vi "Main.vi"() -> ()   [LabVIEW 2013]
uses:
  <vilib>/Utility/error.llb/DialogType.ctl
  <vilib>/Utility/miscctls.llb/LVFontTypeDef.ctl
panel:
  in  "List of channels":i32(listbox)
  in  "ReadFromFile":bool
  in  "WriteToFile":bool
  out "Дата":string
  out "Время":string
  in  "Comm. current inc":dbl=0.5 caption="А" min=0.0 max=72.0 step=0.25
  in  "Common curr. dec":bool
  in  "Common curr. inc":bool
  in  "ConnectAll":bool
  in  "DisconnectAll":bool
  in  "Set Output ON All":bool caption="ВЫХОДЫ ИСТОЧНИКОВ"
  out "текущий ист.":u8
  in  "SetCurrent":dbl min=0.0 max=72.0 step=0.1 format="%#.1g"
  in  "SetVoltage":dbl min=0.0 max=30.0 step=0.1 format="%#.1g"
  in  "SetCurrentB":bool
  in  "SetVoltageB":bool
  in  "SetOutputOffB":bool
  in  "SetOutputOnB":bool
  in  "ConnectChannel":bool
  in  "DisconnectChannel":bool
  in  "stop":bool
  out "Buv con ID":refnum<k5>
  out "LoadPhase":bool
  in  "SetCurrentAll":bool
  in  "SetVoltageAll":bool
  in  "Comm. voltage %":dbl caption="%" min=0.0 max=100.0 step=0.5
  in  "Common volt. dec":bool
  in  "Common volt. inc":bool
  in  "DeleteChannel":bool
  in  "AddChannel":bool
  out "CURRENTSET":dbl[](array[numeric])
  out "NAME":string[](array[string])
  out "ADRESS":string[](array[string])
  out "Measure_VI":refnum<vi>[](array[refnum])
  # "ЛИНЗЫ ЖЕСТКОЙ ФОКУСИРОВКИ ПОСТОЯННОГО ТОКА"
  # "ВСЕ ИСТОЧНИКИ"
  # "ИСТОЧНИК №_"
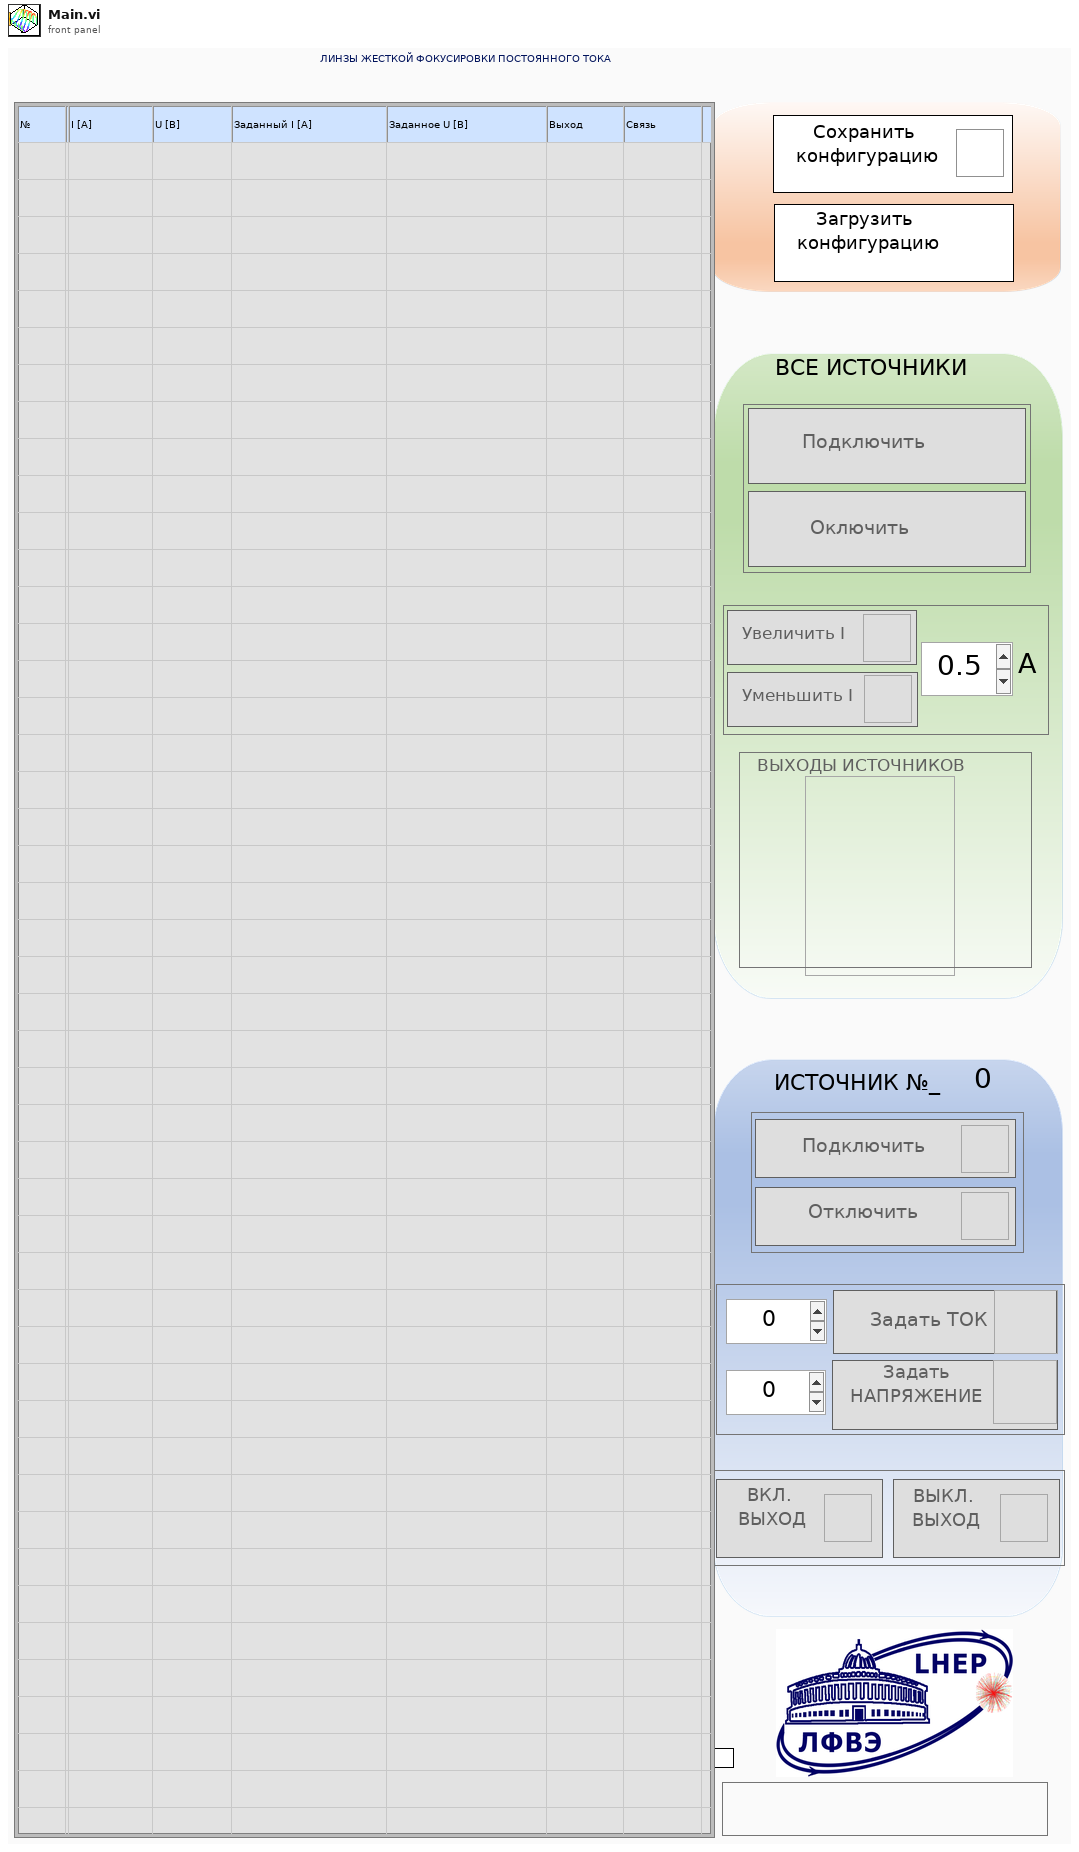
[diagram p1: front panel]
types:
  T1 = enum8{"Enabled", "Disabled", "Disabled and Grayed Out"}
  T2 = enum16{"open", "replace", "create", "open or create", "replace or create", "replace or create with confirmation"}
  T3 = typedef "DialogType.ctl" = u16
  T4 = typedef "LVFontTypeDef.ctl" = cluster{"Font Name":string, "Size":u16, "Bold":bool, "Italic":bool, "Underline":bool, "Strikeout":bool, "Color":u32}
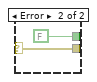
[diagram p7: hidden frame]
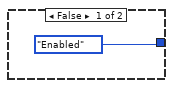
[diagram p9: hidden frame]
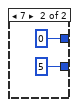
[diagram p11: hidden frame]
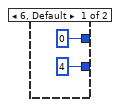
[diagram p12: hidden frame]
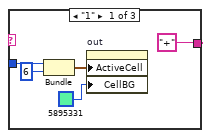
[diagram p13: hidden frame]
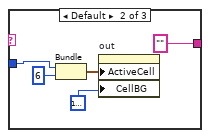
[diagram p14: hidden frame]
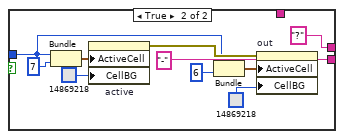
[diagram p15: hidden frame]
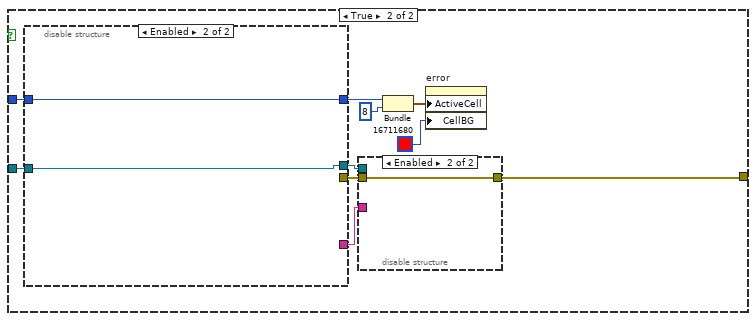
[diagram p16: hidden frame]
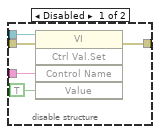
[diagram p17: hidden frame]
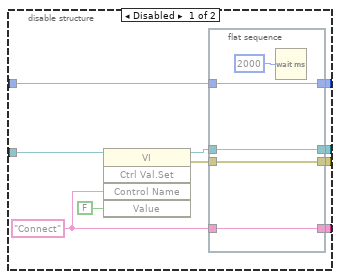
[diagram p18: hidden frame]
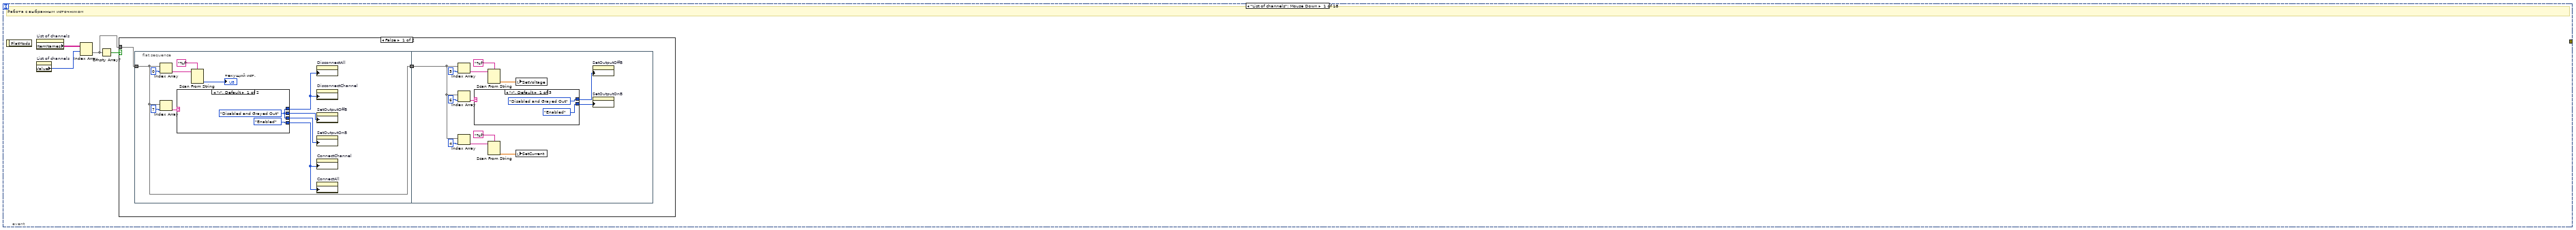
[diagram p19: hidden frame]
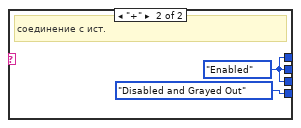
[diagram p20: hidden frame]
diagram:
  w1 = string[] [] ("GlobalInAdress")
  (unwired) T1."Enabled" ("Disabled")
  w17 = u8 0 ("Disabled")
  w4 = FALSE ("SetOutputOnB")
  n1 = while {
    stop <- FALSE stop-if-true
    n2 = property on="List of channels" class="MCListbox (strict)"() -> ("ItemNames"=w29:string[][])  [unwired: 2 in, 2 out]
    n3 = Get Date/Time String(want seconds? (F)=TRUE) -> (date string=→"Дата":string, time string=→"Время":string)  [unwired: 2 in]
    n4 = Wait Until Next ms Multiple(millisecond multiple=u16 1000) -> ()  [unwired: 1 out]
    n5 = Empty Array?(array=w29) -> (empty?=w28:bool)
    n6 = case shown="True" w28 {
      tunnel: [T1."Enabled" ("Disabled") T1."Disabled and Grayed Out" ("Disabled")] -> w23
      frame False {
      }
      frame True {
      }
    }
    n7 = property on="Common curr. inc" class="Bool (strict)"("DisabledEnum"=w23) -> ()  [unwired: 2 in, 2 out]
    n8 = property on="Common curr. dec" class="Bool (strict)"("DisabledEnum"=w23) -> ()  [unwired: 2 in, 2 out]
    n9 = property on="Set Output ON All" class="Bool (strict)"("DisabledEnum"=w23) -> ()  [unwired: 2 in, 2 out]
    n10 = property on="Common volt. inc" class="Bool (strict)"("DisabledEnum"=w23) -> ()  [unwired: 2 in, 2 out]
    n11 = property on="DisconnectAll" class="Bool (strict)"("DisabledEnum"=w23) -> ()  [unwired: 2 in, 2 out]
    n12 = property on="SetVoltageB" class="Bool (strict)"("DisabledEnum"=w23) -> ()  [unwired: 2 in, 2 out]
    n13 = property on="ConnectChannel" class="Bool (strict)"("DisabledEnum"=w23) -> ()  [unwired: 2 in, 2 out]
    n14 = property on="SetOutputOnB" class="Bool (strict)"("DisabledEnum"=w23) -> ()  [unwired: 2 in, 2 out]
    n15 = property on="DisconnectChannel" class="Bool (strict)"("DisabledEnum"=w23) -> ()  [unwired: 2 in, 2 out]
    n16 = property on="SetOutputOffB" class="Bool (strict)"("DisabledEnum"=w23) -> ()  [unwired: 2 in, 2 out]
    n17 = property on="ConnectAll" class="Bool (strict)"("DisabledEnum"=w23) -> ()  [unwired: 2 in, 2 out]
    n18 = property on="SetCurrentB" class="Bool (strict)"("DisabledEnum"=w23) -> ()  [unwired: 2 in, 2 out]
  }
  n19 = while {
    stop <- FALSE stop-if-true
    n20 = property on="AddChannel" class="Bool (strict)"() -> ("Disabled"=w37:u8)  [unwired: 2 in, 2 out]
    n21 = Wait Until Next ms Multiple(millisecond multiple=u32 10) -> ()  [unwired: 1 out]
    n22 = Equal?(x=w37, y=u8 0) -> (x = y?=w33:bool)
    n23 = case shown="True" w33 {
      frame False {
      }
      frame True {
        w43 = string[] [] ("GlobalInAdress")
        n24 = local read "Measure_VI"() -> (w50:refnum<vi>[])
        n25 = Array Size(array=w50) -> (size(s)=w42:i32)
        n26 = for {
          N: w42 -> [_]
          tunnel: w50 -> [w113]
          shift-right: [w55] -> w41
          shift-left: w43 -> [w52]
          shift-right: [w54] -> w40
          shift-left: w43 -> [w53]
          shift-right: [w104] -> w38
          shift-left: w43 -> [w105]
          shift-right: [w95] -> w39
          shift-left: w43 -> [w100]
          shift-right: [w98] -> w46
          shift-left: w43 -> [w80]
          shift-right: [w93] -> w45
          shift-left: w43 -> [w94]
          i -> [w76]
          w92 = "" ("Control Name")
          n27 = Index Array(array=w113, index=w76) -> (element=w79:refnum<vi>)
          n28 = invoke on="Invoke Node" class="VI" method="Ctrl Val.Get"(reference=w79, "Control Name"="SetVoltageStr") -> (error out=w87:errorcluster, "Get Control Value Variant"=w103:variant)  [unwired: 2 in, 2 out]
          n29 = invoke class="VI" method="Ctrl Val.Get"(reference=w79, "Control Name"="SetCurrentStr") -> (error out=w86:errorcluster, "Get Control Value Variant"=w102:variant)  [unwired: 2 in, 2 out]
          n30 = invoke class="VI" method="Ctrl Val.Get"(reference=w79, "Control Name"="Error") -> (error out=w75:errorcluster, "Get Control Value Variant"=w81:variant)  [unwired: 2 in, 2 out]
          n31 = invoke class="VI" method="Ctrl Val.Get"(reference=w79, "Control Name"="GetCurrent") -> (error out=w89:errorcluster, "Get Control Value Variant"=w110:variant)  [unwired: 2 in, 2 out]
          n32 = invoke class="VI" method="Ctrl Val.Get"(reference=w79, "Control Name"="GetVoltage") -> (error out=w88:errorcluster, "Get Control Value Variant"=w111:variant)  [unwired: 2 in, 2 out]
          n33 = invoke class="VI" method="Ctrl Val.Get"(reference=w79, "Control Name"="Output") -> (error out=w85:errorcluster, "Get Control Value Variant"=w96:variant)  [unwired: 2 in, 2 out]
          n34 = Variant To Data(type=w92, Variant=w103) -> (data=w57:string)  [unwired: 1 in, 1 out]
          n35 = Variant To Data(type=w92, Variant=w102) -> (data=w62:string)  [unwired: 1 in, 1 out]
          n36 = Merge Errors(w75, w89, w88, w87) -> (w84:errorcluster)
          n37 = Variant To Data(type=w92, Variant=w110) -> (data=w107:string)  [unwired: 1 in, 1 out]
          n38 = Variant To Data(type=w92, Variant=w111) -> (data=w108:string)  [unwired: 1 in, 1 out]
          n39 = Variant To Data "Out"(type=w92, Variant=w96) -> (data=w82:string)  [unwired: 1 in, 1 out]
          n40 = Merge Errors(w86, w85) -> (w83:errorcluster)
          n41 = String Length(string=w57) -> (length=w58:i32)
          n42 = String Length(string=w62) -> (length=w65:i32)
          n43 = Variant To Data(type=FALSE, Variant=w81) -> (data=w51:bool)  [unwired: 1 in, 1 out]
          n44 = case shown="False" w51 {
            tunnel: w79 -> [_ w167]
            tunnel: w76 -> [w154 w160]
            tunnel: [w153 w158] -> w72
            frame False {
              n45 = Bundle(w154, "milliseconds to wait"=8) -> (w155:cluster{i32, "milliseconds to wait":i32})  [unwired: 1 in]
              n46 = property on="error" class="MCListbox (strict)"("ActiveCell"=w155, "CellBG"=u32 16777225) -> (error out=w153:errorcluster)  [unwired: 2 in, 1 out]
            }
            frame True {
              n47 = disable-structure shown="Enabled" {
                disable-tunnel: w167 -> [w183 w189]
                disable-tunnel: [w180 _] -> w163
                disable-tunnel: [w178 w189] -> w162
                disable-tunnel: [w176 _] -> w161
                disable-tunnel: w160 -> [w175 w190]
                disable-tunnel: [w174 w190] -> w159
                frame Disabled {
                  w177 = "Connect" ("Control Name")
                  n48 = invoke class="VI" method="Ctrl Val.Set"(reference=w183, "Control Name"=w177, "Value"=FALSE ("OK Button")) -> (reference out=w179:refnum<vi>, error out=w181:errorcluster)  [unwired: 2 in, 3 out]
                  n49 = flat-sequence {
                    tunnel: w181 -> [w188]
                    tunnel: [w188] -> w180
                    tunnel: w179 -> [w186]
                    tunnel: [w186] -> w178
                    tunnel: w177 -> [w185]
                    tunnel: [w185] -> w176
                    tunnel: w175 -> [w184]
                    tunnel: [w184] -> w174
                    frame #0 {
                      n50 = Wait (ms)(milliseconds to wait=u32 2000) -> ()  [unwired: 1 out]
                    }
                  }
                }
                frame Enabled {
                }
              }
              n51 = disable-structure shown="Enabled" {
                disable-tunnel: w163 -> [w171 w173]
                disable-tunnel: w162 -> [w170 _]
                disable-tunnel: w161 -> [w169 _]
                disable-tunnel: [w168 w173] -> w158
                frame Disabled {
                  n52 = invoke class="VI" method="Ctrl Val.Set"(reference=w170, error in=w171, "Control Name"=w169, "Value"=TRUE ("OK Button")) -> (error out=w168:errorcluster)  [unwired: 1 in, 4 out]
                }
                frame Enabled {
                }
              }
              n53 = Bundle(w159, "milliseconds to wait"=8) -> (w164:cluster{i32, "milliseconds to wait":i32})  [unwired: 1 in]
              n54 = property on="error" class="MCListbox (strict)"("ActiveCell"=w164, "CellBG"=u32 16711680) -> ()  [unwired: 2 in, 2 out]
            }
          }
          n55 = case shown="6, Default" w58 {
            tunnel: [4 ("milliseconds to wait") 5 ("milliseconds to wait")] -> w59
            tunnel: [0 ("milliseconds to wait") 0 ("milliseconds to wait")] -> w60
            frame 6, Default {
            }
            frame 7 {
            }
          }
          n56 = case shown="7" w65 {
            tunnel: [4 ("milliseconds to wait") 5 ("milliseconds to wait")] -> w64
            tunnel: [0 ("milliseconds to wait") 0 ("milliseconds to wait")] -> w63
            frame 6, Default {
            }
            frame 7 {
            }
          }
          n57 = Build Array (concatenate)(w52, w107) -> (w55:string[])
          n58 = Build Array (concatenate)(w53, w108) -> (w54:string[])
          n59 = Merge Errors(w84, w83, w72) -> (w78:errorcluster)
          n60 = call <vilib>:"General Error Handler.vi"("type of dialog (OK msg:1)"=u32 0 ("milliseconds to wait"), "error in (no error)"=w78) -> ()  [unwired: 9 in, 5 out]
          n61 = case shown="\"0\"" w82 {
            tunnel: ["+" ("Control Name") "" ("Control Name") "-" ("Control Name")] -> w74
            tunnel: w76 -> [w122 w127 w132]
            frame "1" {
              n62 = Bundle(w122, "milliseconds to wait"=6) -> (w124:cluster{i32, "milliseconds to wait":i32})  [unwired: 1 in]
              n63 = property on="out" class="MCListbox (strict)"("ActiveCell"=w124, "CellBG"=u32 5895331) -> ()  [unwired: 2 in, 2 out]
            }
            frame Default {
              n64 = Bundle(w127, "milliseconds to wait"=6) -> (w129:cluster{i32, "milliseconds to wait":i32})  [unwired: 1 in]
              n65 = property on="out" class="MCListbox (strict)"("ActiveCell"=w129, "CellBG"=u32 16777225) -> ()  [unwired: 2 in, 2 out]
            }
            frame "0" {
              n66 = Bundle(w132, "milliseconds to wait"=6) -> (w134:cluster{i32, "milliseconds to wait":i32})  [unwired: 1 in]
              n67 = property on="out" class="MCListbox (strict)"("ActiveCell"=w134, "CellBG"=u32 13816530) -> ()  [unwired: 2 in, 2 out]
            }
          }
          n68 = String Subset(string=w57, offset (0)=w60, length (rest)=w59) -> (substring=w56:string)
          n69 = String Subset(string=w62, offset (0)=w63, length (rest)=w64) -> (substring=w61:string)
          n70 = case shown="False" w51 {
            tunnel: ["+" ("Control Name") "-" ("Control Name")] -> w99
            tunnel: w76 -> [w138 w145]
            tunnel: w74 -> [w137 _]
            tunnel: [w137 "?" ("Control Name")] -> w73
            frame False {
              n71 = Bundle(w138, "milliseconds to wait"=7) -> (w140:cluster{i32, "milliseconds to wait":i32})  [unwired: 1 in]
              n72 = property on="active" class="MCListbox (strict)"("ActiveCell"=w140, "CellBG"=u32 5895331) -> ()  [unwired: 2 in, 2 out]
            }
            frame True {
              n73 = Bundle(w145, "milliseconds to wait"=7) -> (w151:cluster{i32, "milliseconds to wait":i32})  [unwired: 1 in]
              n74 = property on="active" class="MCListbox (strict)"("ActiveCell"=w151, "CellBG"=u32 14869218) -> (error out=w146:errorcluster)  [unwired: 2 in, 1 out]
              n75 = Bundle(w145, "milliseconds to wait"=6) -> (w144:cluster{i32, "milliseconds to wait":i32})  [unwired: 1 in]
              n76 = property on="out" class="MCListbox (strict)"(error in=w146, "ActiveCell"=w144, "CellBG"=u32 14869218) -> ()  [unwired: 1 in, 2 out]
            }
          }
          n77 = Search and Replace String(input string=w56, search string=",", replace string="." ("replace string (\"\")")) -> (result string=w69:string)  [unwired: 5 in, 3 out]
          n78 = Search and Replace String(input string=w61, search string=",", replace string="." ("replace string (\"\")")) -> (result string=w67:string)  [unwired: 5 in, 3 out]
          n79 = Build Array (concatenate)(w100, w67) -> (w95:string[])
          n80 = Build Array (concatenate)(w105, w69) -> (w104:string[])
          n81 = Build Array (concatenate)(w94, w73) -> (w93:string[])
          n82 = Build Array (concatenate)(w80, w99) -> (w98:string[])
        }
        n83 = local read "ADRESS"() -> (w48:string[])
        n84 = local read "NAME"() -> (w47:string[])
        n85 = Build Array(w47, w48, w41, w40, w39, w38, w45, w46) -> (w49:string[][])
        n86 = Transpose 2D Array(2D array=w49) -> (transposed array=w44:string[][])
        n87 = property on="List of channels" class="MCListbox (strict)"("ItemNames"=w44) -> ()  [unwired: 2 in, 2 out]
      }
    }
  }
  n88 = while {
    stop <- FALSE stop-if-true
    n89 = event shown="[11] \"SetOutputOnB\": Value Change" {
      selector: _ -> [_ _ _ _ _ _ _ _ _ _ _ _ _ _ _ _ _ _]
      dyn-events: _ -> [_ _ _ _ _ _ _ _ _ _ _ _ _ _ _ _ _ _]
      timeout: _ -> [_ _ _ _ _ _ _ _ _ _ _ _ _ _ _ _ _ _]
      tunnel: [_ _ w261 w277 w293 w334 w375 w390 w421 w437 w453 w470 w491 w514 w532 w583 w661 w684] -> w192
      event "List of channels": Mouse Down {
        # "Работа с выбранным источником"
        n90 = event-data() -> ()  [unwired: 2 out]
        n91 = property on="List of channels" class="MCListbox (strict)"() -> ("ItemNames"=w198:string[][])  [unwired: 2 in, 2 out]
        n92 = property on="List of channels" class="MCListbox (strict)"() -> ("Value"=w197:i32)  [unwired: 2 in, 2 out]
        n93 = Index Array(array=w198, index (row)=w197) -> (element=w196:string[])  [unwired: 1 in]
        n94 = Empty Array?(array=w196) -> (empty?=w195:bool)
        n95 = case shown="False" w195 {
          tunnel: w196 -> [w199 _]
          frame False {
            n96 = flat-sequence {
              tunnel: w199 -> [w205]
              tunnel: [w205] -> w200
              tunnel: w200 -> [w218]
              frame #0 {
                n97 = Index Array(array=w205, index=0) -> (element=w208:string)
                n98 = Index Array(array=w205, index=7) -> (element=w206:string)
                n99 = case shown="\"-\", Default" w206 {
                  tunnel: [T1."Enabled" ("Disabled") T1."Disabled and Grayed Out" ("Disabled")] -> w201
                  tunnel: [w212 w214] -> w202
                  tunnel: [w212 w214] -> w204
                  tunnel: [w212 w214] -> w203
                  frame "-", Default {
                    w212 = T1."Disabled and Grayed Out" ("Disabled")
                  }
                  frame "+" {
                    w214 = T1."Enabled" ("Disabled")
                    # "соединение с ист."
                  }
                }
                n100 = Scan From String(format string="%f", input string=w208) -> (output 1=→"текущий ист.":u8)  [unwired: 3 in, 3 out]
                n101 = property on="DisconnectAll" class="Bool (strict)"("DisabledEnum"=w202) -> ()  [unwired: 2 in, 2 out]
                n102 = property on="DisconnectChannel" class="Bool (strict)"("DisabledEnum"=w202) -> ()  [unwired: 2 in, 2 out]
                n103 = property on="SetOutputOffB" class="Bool (strict)"("DisabledEnum"=w204) -> ()  [unwired: 2 in, 2 out]
                n104 = property on="SetOutputOnB" class="Bool (strict)"("DisabledEnum"=w203) -> ()  [unwired: 2 in, 2 out]
                n105 = property on="ConnectChannel" class="Bool (strict)"("DisabledEnum"=w201) -> ()  [unwired: 2 in, 2 out]
                n106 = property on="ConnectAll" class="Bool (strict)"("DisabledEnum"=w201) -> ()  [unwired: 2 in, 2 out]
              }
              frame #1 {
                n107 = Index Array(array=w218, index=5) -> (element=w223:string)
                n108 = Index Array(array=w218, index=6) -> (element=w226:string)
                n109 = Index Array(array=w218, index=4) -> (element=w220:string)
                n110 = case shown="\"-\", Default" w226 {
                  tunnel: [T1."Enabled" ("Disabled") T1."Disabled and Grayed Out" ("Disabled") w233] -> w227
                  tunnel: [T1."Disabled and Grayed Out" ("Disabled") T1."Enabled" ("Disabled") w233] -> w228
                  frame "-", Default {
                  }
                  frame "+" {
                  }
                  frame "?" {
                    w233 = T1."Disabled and Grayed Out" ("Disabled")
                  }
                }
                n111 = Scan From String(format string="%f", input string=w223) -> (output 1=w216:dbl)  [unwired: 3 in, 3 out]
                n112 = Scan From String(format string="%f", input string=w220) -> (output 1=w217:dbl)  [unwired: 3 in, 3 out]
                n113 = local write "SetVoltage"(w216) -> ()
                n114 = local write "SetCurrent"(w217) -> ()
                n115 = property on="SetOutputOffB" class="Bool (strict)"("DisabledEnum"=w228) -> ()  [unwired: 2 in, 2 out]
                n116 = property on="SetOutputOnB" class="Bool (strict)"("DisabledEnum"=w227) -> ()  [unwired: 2 in, 2 out]
              }
            }
          }
          frame True {
          }
        }
      }
      event Panel Close? {
        n117 = event-data() -> ()  [unwired: 5 out]
        n118 = Two Button Dialog(message="Вы уверены, что хотите закрыть программу?", 1:"Нет" ("F button name (\"Cancel\")"), 2:"Да" ("T button name (\"OK\")")) -> (T button?=w237:bool)
        n119 = case shown="True" w237 {
          frame False {
          }
          frame True {
            n120 = disable-structure shown="Disabled" {
              frame Disabled {
                n121 = local read item#-1() -> (w247)
                n122 = TCP Close Connection(connection ID=w247) -> ()  [unwired: 2 in, 2 out]
              }
              frame Enabled {
              }
            }
            n123 = local read "Measure_VI"() -> (w239:refnum<vi>[])
            n124 = Array Size(array=w239) -> (size(s)=w238:i32)
            n125 = for {
              N: w238 -> [_]
              tunnel: w239 -> [w257]
              tunnel: [w255] -> w246 mode=indexing
              i -> [w258]
              n126 = Index Array(array=w257, index=w258) -> (element=w256:refnum<vi>)
              n127 = invoke class="VI" method="Ctrl Val.Set"(reference=w256, "Control Name"="Connect", "Value"=FALSE) -> (error out=w255:errorcluster)  [unwired: 2 in, 4 out]
            }
            n128 = flat-sequence {
              tunnel: [w249] -> w245
              tunnel: w246 -> [w249]
              frame #0 {
                n129 = Wait (ms)(milliseconds to wait=u32 1000) -> ()  [unwired: 1 out]
              }
            }
            n130 = local read "Measure_VI"() -> (w240:refnum<vi>[])
            n131 = Array Size(array=w240) -> (size(s)=w241:i32)
            n132 = for {
              N: w241 -> [_]
              tunnel: w240 -> [w253]
              tunnel: [w251] -> w242 mode=indexing
              tunnel: w245 -> [w250] mode=indexing
              i -> [w254]
              n133 = Index Array(array=w253, index=w254) -> (element=w252:refnum<vi>)
              n134 = invoke class="VI" method="Abort VI"(reference=w252, error in=w250) -> (error out=w251:errorcluster)  [unwired: 1 in, 2 out]
            }
            n135 = Merge Errors(w242) -> (w243:errorcluster)
            n136 = call <vilib>:"General Error Handler.vi"("type of dialog (OK msg:1)"=u32 0 ("milliseconds to wait"), "error in (no error)"=w243) -> ()  [unwired: 9 in, 5 out]
          }
        }
        n137 = event-data() -> ()  [unwired: 2 in, 1 out]
      }
      event "SetVoltageAll": Value Change {
        n138 = event-data() -> ()  [unwired: 7 out]
        n139 = flat-sequence {
          tunnel: [w265] -> w263
          tunnel: [w274] -> w262
          tunnel: w263 -> [w274]
          frame #0 {
            w264 = u8 2 ("Disabled")
            n140 = property on="AddChannel" class="Bool (strict)"("Disabled"=w264) -> ()  [unwired: 2 in, 2 out]
            n141 = property on="DisconnectChannel" class="Bool (strict)"("Disabled"=w264) -> ()  [unwired: 2 in, 2 out]
            n142 = property on="ConnectAll" class="Bool (strict)"("Disabled"=w264) -> ()  [unwired: 2 in, 2 out]
            n143 = property on="ReadFromFile" class="Bool (strict)"("Disabled"=w264) -> ()  [unwired: 2 in, 2 out]
            n144 = property on="ConnectChannel" class="Bool (strict)"("Disabled"=w264) -> ()  [unwired: 2 in, 2 out]
            n145 = property on="DeleteChannel" class="Bool (strict)"("Disabled"=w264) -> ()  [unwired: 2 in, 2 out]
            n146 = property on="SetVoltageB" class="Bool (strict)"("Disabled"=w264) -> ()  [unwired: 2 in, 2 out]
            n147 = property on="Set Output ON All" class="Bool (strict)"("Disabled"=w264) -> ()  [unwired: 2 in, 2 out]
            n148 = property on="SetOutputOffB" class="Bool (strict)"("Disabled"=w264) -> ()  [unwired: 2 in, 2 out]
            n149 = property on="SetVoltageAll" class="Bool (strict)"("Disabled"=w264) -> ()  [unwired: 2 in, 2 out]
            n150 = property on="SetCurrentAll" class="Bool (strict)"("Disabled"=w264) -> ()  [unwired: 2 in, 2 out]
            n151 = property on="DisconnectAll" class="Bool (strict)"("Disabled"=w264) -> ()  [unwired: 2 in, 2 out]
            n152 = property on="WriteToFile" class="Bool (strict)"("Disabled"=w264) -> ()  [unwired: 2 in, 2 out]
            n153 = property on="SetCurrentB" class="Bool (strict)"("Disabled"=w264) -> ()  [unwired: 2 in, 2 out]
            n154 = property on="SetOutputOnB" class="Bool (strict)"("Disabled"=w264) -> ()  [unwired: 2 in, 2 out]
          }
          frame #1 {
            n155 = local read "Measure_VI"() -> (w267:refnum<vi>[])
            n156 = Array Size(array=w267) -> (size(s)=w266:i32)
            n157 = for {
              N: w266 -> [_]
              tunnel: [w268] -> w265 mode=indexing
              i -> [w270]
              n158 = local read "Measure_VI"() -> (w273:refnum<vi>[])
              n159 = Index Array(array=w273, index=w270) -> (element=w269:refnum<vi>)
              n160 = invoke class="VI" method="Ctrl Val.Set"(reference=w269, "Control Name"="NeedToSetVoltage", "Value"=TRUE ("ConnectChannel")) -> (error out=w268:errorcluster)  [unwired: 2 in, 4 out]
            }
          }
          frame #2 {
            w275 = u8 0 ("Disabled")
            n161 = local write "SetVoltageAll"(FALSE ("SetVoltageAll")) -> ()
            n162 = property on="AddChannel" class="Bool (strict)"("Disabled"=w275) -> ()  [unwired: 2 in, 2 out]
            n163 = property on="DisconnectChannel" class="Bool (strict)"("Disabled"=w275) -> ()  [unwired: 2 in, 2 out]
            n164 = property on="ReadFromFile" class="Bool (strict)"("Disabled"=w275) -> ()  [unwired: 2 in, 2 out]
            n165 = property on="ConnectChannel" class="Bool (strict)"("Disabled"=w275) -> ()  [unwired: 2 in, 2 out]
            n166 = property on="DeleteChannel" class="Bool (strict)"("Disabled"=w275) -> ()  [unwired: 2 in, 2 out]
            n167 = property on="WriteToFile" class="Bool (strict)"("Disabled"=w275) -> ()  [unwired: 2 in, 2 out]
            n168 = property on="Set Output ON All" class="Bool (strict)"("Disabled"=w275) -> ()  [unwired: 2 in, 2 out]
            n169 = property on="SetCurrentB" class="Bool (strict)"("Disabled"=w275) -> ()  [unwired: 2 in, 2 out]
            n170 = property on="ConnectAll" class="Bool (strict)"("Disabled"=w275) -> ()  [unwired: 2 in, 2 out]
            n171 = property on="SetOutputOnB" class="Bool (strict)"("Disabled"=w275) -> ()  [unwired: 2 in, 2 out]
            n172 = property on="SetVoltageB" class="Bool (strict)"("Disabled"=w275) -> ()  [unwired: 2 in, 2 out]
            n173 = property on="SetOutputOffB" class="Bool (strict)"("Disabled"=w275) -> ()  [unwired: 2 in, 2 out]
            n174 = property on="SetVoltageAll" class="Bool (strict)"("Disabled"=w275) -> ()  [unwired: 2 in, 2 out]
            n175 = property on="SetCurrentAll" class="Bool (strict)"("Disabled"=w275) -> ()  [unwired: 2 in, 2 out]
            n176 = property on="DisconnectAll" class="Bool (strict)"("Disabled"=w275) -> ()  [unwired: 2 in, 2 out]
          }
        }
        n177 = Merge Errors(w262) -> (w261:errorcluster)
      }
      event "SetCurrentAll": Value Change {
        n178 = event-data() -> ()  [unwired: 7 out]
        n179 = flat-sequence {
          tunnel: [w281] -> w279
          tunnel: [w290] -> w278
          tunnel: w279 -> [w290]
          frame #0 {
            w280 = u8 2 ("Disabled")
            n180 = property on="AddChannel" class="Bool (strict)"("Disabled"=w280) -> ()  [unwired: 2 in, 2 out]
            n181 = property on="DisconnectChannel" class="Bool (strict)"("Disabled"=w280) -> ()  [unwired: 2 in, 2 out]
            n182 = property on="ConnectAll" class="Bool (strict)"("Disabled"=w280) -> ()  [unwired: 2 in, 2 out]
            n183 = property on="ReadFromFile" class="Bool (strict)"("Disabled"=w280) -> ()  [unwired: 2 in, 2 out]
            n184 = property on="ConnectChannel" class="Bool (strict)"("Disabled"=w280) -> ()  [unwired: 2 in, 2 out]
            n185 = property on="DeleteChannel" class="Bool (strict)"("Disabled"=w280) -> ()  [unwired: 2 in, 2 out]
            n186 = property on="SetOutputOffB" class="Bool (strict)"("Disabled"=w280) -> ()  [unwired: 2 in, 2 out]
            n187 = property on="Set Output ON All" class="Bool (strict)"("Disabled"=w280) -> ()  [unwired: 2 in, 2 out]
            n188 = property on="SetVoltageAll" class="Bool (strict)"("Disabled"=w280) -> ()  [unwired: 2 in, 2 out]
            n189 = property on="SetCurrentAll" class="Bool (strict)"("Disabled"=w280) -> ()  [unwired: 2 in, 2 out]
            n190 = property on="DisconnectAll" class="Bool (strict)"("Disabled"=w280) -> ()  [unwired: 2 in, 2 out]
            n191 = property on="WriteToFile" class="Bool (strict)"("Disabled"=w280) -> ()  [unwired: 2 in, 2 out]
            n192 = property on="SetCurrentB" class="Bool (strict)"("Disabled"=w280) -> ()  [unwired: 2 in, 2 out]
            n193 = property on="SetOutputOnB" class="Bool (strict)"("Disabled"=w280) -> ()  [unwired: 2 in, 2 out]
            n194 = property on="SetVoltageB" class="Bool (strict)"("Disabled"=w280) -> ()  [unwired: 2 in, 2 out]
          }
          frame #1 {
            n195 = local read "Measure_VI"() -> (w283:refnum<vi>[])
            n196 = Array Size(array=w283) -> (size(s)=w282:i32)
            n197 = for {
              N: w282 -> [_]
              tunnel: [w284] -> w281 mode=indexing
              i -> [w286]
              n198 = local read "Measure_VI"() -> (w289:refnum<vi>[])
              n199 = Index Array(array=w289, index=w286) -> (element=w285:refnum<vi>)
              n200 = invoke class="VI" method="Ctrl Val.Set"(reference=w285, "Control Name"="NeedToSetCurrent", "Value"=TRUE ("ConnectChannel")) -> (error out=w284:errorcluster)  [unwired: 2 in, 4 out]
            }
          }
          frame #2 {
            w291 = u8 0 ("Disabled")
            n201 = local write "SetCurrentAll"(FALSE ("SetVoltageAll")) -> ()
            n202 = property on="AddChannel" class="Bool (strict)"("Disabled"=w291) -> ()  [unwired: 2 in, 2 out]
            n203 = property on="DisconnectChannel" class="Bool (strict)"("Disabled"=w291) -> ()  [unwired: 2 in, 2 out]
            n204 = property on="ReadFromFile" class="Bool (strict)"("Disabled"=w291) -> ()  [unwired: 2 in, 2 out]
            n205 = property on="ConnectChannel" class="Bool (strict)"("Disabled"=w291) -> ()  [unwired: 2 in, 2 out]
            n206 = property on="DeleteChannel" class="Bool (strict)"("Disabled"=w291) -> ()  [unwired: 2 in, 2 out]
            n207 = property on="WriteToFile" class="Bool (strict)"("Disabled"=w291) -> ()  [unwired: 2 in, 2 out]
            n208 = property on="Set Output ON All" class="Bool (strict)"("Disabled"=w291) -> ()  [unwired: 2 in, 2 out]
            n209 = property on="SetCurrentB" class="Bool (strict)"("Disabled"=w291) -> ()  [unwired: 2 in, 2 out]
            n210 = property on="ConnectAll" class="Bool (strict)"("Disabled"=w291) -> ()  [unwired: 2 in, 2 out]
            n211 = property on="SetOutputOnB" class="Bool (strict)"("Disabled"=w291) -> ()  [unwired: 2 in, 2 out]
            n212 = property on="SetVoltageB" class="Bool (strict)"("Disabled"=w291) -> ()  [unwired: 2 in, 2 out]
            n213 = property on="SetOutputOffB" class="Bool (strict)"("Disabled"=w291) -> ()  [unwired: 2 in, 2 out]
            n214 = property on="SetVoltageAll" class="Bool (strict)"("Disabled"=w291) -> ()  [unwired: 2 in, 2 out]
            n215 = property on="SetCurrentAll" class="Bool (strict)"("Disabled"=w291) -> ()  [unwired: 2 in, 2 out]
            n216 = property on="DisconnectAll" class="Bool (strict)"("Disabled"=w291) -> ()  [unwired: 2 in, 2 out]
          }
        }
        n217 = Merge Errors(w278) -> (w277:errorcluster)
      }
      event "Common curr. inc", "Common curr. dec": Value Change {
        # "Увелич/уменьшение тока на всех ист"
        n218 = event-data() -> ()  [unwired: 2 out]
        n219 = local read "ADRESS"() -> (w296:string[])
        n220 = Array Size(array=w296) -> (size(s)=w297:i32)
        n221 = for {
          N: w297 -> [_]
          tunnel: [w307] -> w295 mode=indexing
          i -> [w321]
          n222 = local read "Measure_VI"() -> (w324:refnum<vi>[])
          n223 = Index Array(array=w324, index=w321) -> (element=w315:refnum<vi>)
          n224 = invoke class="VI" method="Ctrl Val.Get"(reference=w315, "Control Name"="SetCurrentStr") -> (reference out=w309:refnum<vi>, error out=w319:errorcluster, "Get Control Value Variant"=w323:variant)  [unwired: 2 in, 1 out]
          n225 = Variant To Data(error in=w319, type="" ("Control Name"), Variant=w323) -> (data=w318:string, error out=w317:errorcluster)
          n226 = Scan From String(format string="%f", input string=w318, error in=w317) -> (error out=w308:errorcluster, output 1=w306:dbl)  [unwired: 2 in, 2 out]
          n227 = local read "Common curr. inc"() -> (w305:bool)
          n228 = local read "Common curr. dec"() -> (w303:bool)
          n229 = case shown="True" w305 {
            tunnel: "Comm. current inc" -> [w329 w333]
            tunnel: w306 -> [w330 w332]
            tunnel: [w330 w331] -> w304
            tunnel: [w329 _] -> w302
            frame False {
            }
            frame True {
              n230 = Add(x=w332, y=w333) -> (x+y=w331:dbl)
            }
          }
          n231 = case shown="True" w303 {
            tunnel: w304 -> [w325 w328]
            tunnel: [w325 w327] -> w301
            tunnel: w302 -> [_ w326]
            frame False {
            }
            frame True {
              n232 = Subtract(x=w328, y=w326) -> (x-y=w327:dbl)
            }
          }
          n233 = invoke class="VI" method="Ctrl Val.Set"(reference=w309, error in=w308, "Control Name"="SetCurrent", "Value"=w301) -> (reference out=w311:refnum<vi>, error out=w310:errorcluster)  [unwired: 1 in, 3 out]
          n234 = invoke class="VI" method="Ctrl Val.Set"(reference=w311, error in=w310, "Control Name"="NeedToSetCurrent", "Value"=TRUE ("ConnectChannel")) -> (error out=w307:errorcluster)  [unwired: 1 in, 4 out]
        }
        n235 = Merge Errors(w295) -> (w294:errorcluster)
        n236 = flat-sequence {
          tunnel: w294 -> [w299]
          tunnel: [w299] -> w293
          frame #0 {
            w298 = FALSE ("ConnectChannel")
            n237 = local write "Common curr. inc"(w298) -> ()
            n238 = local write "Common curr. dec"(w298) -> ()
          }
        }
      }
      event "Common volt. inc", "Common volt. dec": Value Change {
        # "Увелич/уменьшение тока на всех ист"
        n239 = event-data() -> ()  [unwired: 2 out]
        n240 = local read "ADRESS"() -> (w337:string[])
        n241 = Array Size(array=w337) -> (size(s)=w338:i32)
        n242 = for {
          N: w338 -> [_]
          tunnel: [w348] -> w336 mode=indexing
          i -> [w362]
          n243 = local read "Measure_VI"() -> (w365:refnum<vi>[])
          n244 = Index Array(array=w365, index=w362) -> (element=w356:refnum<vi>)
          n245 = invoke class="VI" method="Ctrl Val.Get"(reference=w356, "Control Name"="SetVoltageStr") -> (reference out=w350:refnum<vi>, error out=w360:errorcluster, "Get Control Value Variant"=w364:variant)  [unwired: 2 in, 1 out]
          n246 = Variant To Data(error in=w360, type="" ("Control Name"), Variant=w364) -> (data=w359:string, error out=w358:errorcluster)
          n247 = Scan From String(format string="%f", input string=w359, error in=w358) -> (error out=w349:errorcluster, output 1=w347:dbl)  [unwired: 2 in, 2 out]
          n248 = local read "Common volt. inc"() -> (w346:bool)
          n249 = local read "Common volt. dec"() -> (w344:bool)
          n250 = case shown="True" w346 {
            tunnel: "Comm. voltage %" -> [w370 w374]
            tunnel: w347 -> [w371 w373]
            tunnel: [w371 w372] -> w345
            tunnel: [w370 _] -> w343
            frame False {
            }
            frame True {
              n251 = Add(x=w373, y=w374) -> (x+y=w372:dbl)
            }
          }
          n252 = case shown="False" w344 {
            tunnel: w345 -> [w366 w369]
            tunnel: [w366 w368] -> w342
            tunnel: w343 -> [_ w367]
            frame False {
            }
            frame True {
              n253 = Subtract(x=w369, y=w367) -> (x-y=w368:dbl)
            }
          }
          n254 = invoke class="VI" method="Ctrl Val.Set"(reference=w350, error in=w349, "Control Name"="SetVoltage", "Value"=w342) -> (reference out=w352:refnum<vi>, error out=w351:errorcluster)  [unwired: 1 in, 3 out]
          n255 = invoke class="VI" method="Ctrl Val.Set"(reference=w352, error in=w351, "Control Name"="NeedToSetVoltage", "Value"=TRUE ("ConnectChannel")) -> (error out=w348:errorcluster)  [unwired: 1 in, 4 out]
        }
        n256 = Merge Errors(w336) -> (w335:errorcluster)
        n257 = flat-sequence {
          tunnel: w335 -> [w340]
          tunnel: [w340] -> w334
          frame #0 {
            w339 = FALSE ("ConnectChannel")
            n258 = local write "Common volt. inc"(w339) -> ()
            n259 = local write "Common volt. dec"(w339) -> ()
          }
        }
      }
      event "DisconnectChannel": Value Change {
        n260 = event-data() -> ()  [unwired: 7 out]
        n261 = property on="List of channels" class="MCListbox (strict)"() -> ("Value"=w379:i32)  [unwired: 2 in, 2 out]
        n262 = flat-sequence {
          tunnel: w379 -> [w381]
          tunnel: [w381] -> w378
          tunnel: w378 -> [w383]
          tunnel: [w382] -> w376
          tunnel: [w388] -> w377
          tunnel: w376 -> [w388]
          frame #0 {
            w380 = u8 2 ("Disabled")
            n263 = property on="AddChannel" class="Bool (strict)"("Disabled"=w380) -> ()  [unwired: 2 in, 2 out]
            n264 = property on="Set Output ON All" class="Bool (strict)"("Disabled"=w380) -> ()  [unwired: 2 in, 2 out]
            n265 = property on="ConnectAll" class="Bool (strict)"("Disabled"=w380) -> ()  [unwired: 2 in, 2 out]
            n266 = property on="DisconnectChannel" class="Bool (strict)"("Disabled"=w380) -> ()  [unwired: 2 in, 2 out]
            n267 = property on="ReadFromFile" class="Bool (strict)"("Disabled"=w380) -> ()  [unwired: 2 in, 2 out]
            n268 = property on="ConnectChannel" class="Bool (strict)"("Disabled"=w380) -> ()  [unwired: 2 in, 2 out]
            n269 = property on="DeleteChannel" class="Bool (strict)"("Disabled"=w380) -> ()  [unwired: 2 in, 2 out]
            n270 = property on="WriteToFile" class="Bool (strict)"("Disabled"=w380) -> ()  [unwired: 2 in, 2 out]
            n271 = property on="SetCurrentB" class="Bool (strict)"("Disabled"=w380) -> ()  [unwired: 2 in, 2 out]
            n272 = property on="SetOutputOnB" class="Bool (strict)"("Disabled"=w380) -> ()  [unwired: 2 in, 2 out]
            n273 = property on="SetVoltageB" class="Bool (strict)"("Disabled"=w380) -> ()  [unwired: 2 in, 2 out]
            n274 = property on="SetOutputOffB" class="Bool (strict)"("Disabled"=w380) -> ()  [unwired: 2 in, 2 out]
            n275 = property on="SetVoltageAll" class="Bool (strict)"("Disabled"=w380) -> ()  [unwired: 2 in, 2 out]
            n276 = property on="SetCurrentAll" class="Bool (strict)"("Disabled"=w380) -> ()  [unwired: 2 in, 2 out]
            n277 = property on="DisconnectAll" class="Bool (strict)"("Disabled"=w380) -> ()  [unwired: 2 in, 2 out]
          }
          frame #1 {
            w384 = FALSE ("OK Button")
            n278 = local write "DisconnectChannel"(w384) -> ()
            n279 = local read "Measure_VI"() -> (w386:refnum<vi>[])
            n280 = Index Array(array=w386, index=w383) -> (element=w385:refnum<vi>)
            n281 = invoke class="VI" method="Ctrl Val.Set"(reference=w385, "Control Name"="Connect", "Value"=w384) -> (error out=w382:errorcluster)  [unwired: 2 in, 4 out]
          }
          frame #2 {
            w389 = u8 0 ("Disabled")
            n282 = property on="AddChannel" class="Bool (strict)"("Disabled"=w389) -> ()  [unwired: 2 in, 2 out]
            n283 = property on="DisconnectChannel" class="Bool (strict)"("Disabled"=w389) -> ()  [unwired: 2 in, 2 out]
            n284 = property on="ConnectAll" class="Bool (strict)"("Disabled"=w389) -> ()  [unwired: 2 in, 2 out]
            n285 = property on="ReadFromFile" class="Bool (strict)"("Disabled"=w389) -> ()  [unwired: 2 in, 2 out]
            n286 = property on="ConnectChannel" class="Bool (strict)"("Disabled"=w389) -> ()  [unwired: 2 in, 2 out]
            n287 = property on="DeleteChannel" class="Bool (strict)"("Disabled"=w389) -> ()  [unwired: 2 in, 2 out]
            n288 = property on="SetOutputOffB" class="Bool (strict)"("Disabled"=w389) -> ()  [unwired: 2 in, 2 out]
            n289 = property on="Set Output ON All" class="Bool (strict)"("Disabled"=w389) -> ()  [unwired: 2 in, 2 out]
            n290 = property on="SetVoltageAll" class="Bool (strict)"("Disabled"=w389) -> ()  [unwired: 2 in, 2 out]
            n291 = property on="SetCurrentAll" class="Bool (strict)"("Disabled"=w389) -> ()  [unwired: 2 in, 2 out]
            n292 = property on="DisconnectAll" class="Bool (strict)"("Disabled"=w389) -> ()  [unwired: 2 in, 2 out]
            n293 = property on="WriteToFile" class="Bool (strict)"("Disabled"=w389) -> ()  [unwired: 2 in, 2 out]
            n294 = property on="SetCurrentB" class="Bool (strict)"("Disabled"=w389) -> ()  [unwired: 2 in, 2 out]
            n295 = property on="SetOutputOnB" class="Bool (strict)"("Disabled"=w389) -> ()  [unwired: 2 in, 2 out]
            n296 = property on="SetVoltageB" class="Bool (strict)"("Disabled"=w389) -> ()  [unwired: 2 in, 2 out]
          }
        }
        n297 = Merge Errors(w377) -> (w375:errorcluster)
      }
      event "ConnectChannel": Value Change {
        n298 = event-data() -> ()  [unwired: 7 out]
        n299 = property on="List of channels" class="MCListbox (strict)"() -> ("Value"=w394:i32)  [unwired: 2 in, 2 out]
        n300 = flat-sequence {
          tunnel: w394 -> [w396]
          tunnel: [w396] -> w393
          tunnel: w393 -> [w403]
          tunnel: [w402] -> w391
          tunnel: [w418] -> w392
          tunnel: w391 -> [w418]
          frame #0 {
            w395 = u8 2 ("Disabled")
            n301 = property on="AddChannel" class="Bool (strict)"("Disabled"=w395) -> ()  [unwired: 2 in, 2 out]
            n302 = property on="Set Output ON All" class="Bool (strict)"("Disabled"=w395) -> ()  [unwired: 2 in, 2 out]
            n303 = property on="ConnectAll" class="Bool (strict)"("Disabled"=w395) -> ()  [unwired: 2 in, 2 out]
            n304 = property on="DisconnectChannel" class="Bool (strict)"("Disabled"=w395) -> ()  [unwired: 2 in, 2 out]
            n305 = property on="ReadFromFile" class="Bool (strict)"("Disabled"=w395) -> ()  [unwired: 2 in, 2 out]
            n306 = property on="ConnectChannel" class="Bool (strict)"("Disabled"=w395) -> ()  [unwired: 2 in, 2 out]
            n307 = property on="DeleteChannel" class="Bool (strict)"("Disabled"=w395) -> ()  [unwired: 2 in, 2 out]
            n308 = property on="WriteToFile" class="Bool (strict)"("Disabled"=w395) -> ()  [unwired: 2 in, 2 out]
            n309 = property on="SetCurrentB" class="Bool (strict)"("Disabled"=w395) -> ()  [unwired: 2 in, 2 out]
            n310 = property on="SetOutputOnB" class="Bool (strict)"("Disabled"=w395) -> ()  [unwired: 2 in, 2 out]
            n311 = property on="SetVoltageB" class="Bool (strict)"("Disabled"=w395) -> ()  [unwired: 2 in, 2 out]
            n312 = property on="SetOutputOffB" class="Bool (strict)"("Disabled"=w395) -> ()  [unwired: 2 in, 2 out]
            n313 = property on="SetVoltageAll" class="Bool (strict)"("Disabled"=w395) -> ()  [unwired: 2 in, 2 out]
            n314 = property on="SetCurrentAll" class="Bool (strict)"("Disabled"=w395) -> ()  [unwired: 2 in, 2 out]
            n315 = property on="DisconnectAll" class="Bool (strict)"("Disabled"=w395) -> ()  [unwired: 2 in, 2 out]
          }
          frame #1 {
            n316 = local read "Measure_VI"() -> (w404:refnum<vi>[])
            n317 = Index Array(array=w404, index=w403) -> (element=w401:refnum<vi>)
            n318 = flat-sequence {
              tunnel: w401 -> [w407]
              tunnel: [w406] -> w399
              tunnel: [w405] -> w397
              tunnel: [w411] -> w400
              tunnel: w399 -> [w411]
              tunnel: [w410] -> w398
              tunnel: w397 -> [w410]
              tunnel: [w414] -> w402
              tunnel: w400 -> [w415]
              tunnel: w398 -> [w413]
              frame #0 {
                n319 = invoke class="VI" method="Ctrl Val.Set"(reference=w407, "Control Name"="Connect", "Value"=FALSE ("OK Button")) -> (reference out=w406:refnum<vi>, error out=w405:errorcluster)  [unwired: 2 in, 3 out]
              }
              frame #1 {
                n320 = Wait (ms)(milliseconds to wait=u32 1000) -> ()  [unwired: 1 out]
              }
              frame #2 {
                n321 = invoke class="VI" method="Ctrl Val.Set"(reference=w415, error in=w413, "Control Name"="Connect", "Value"=TRUE ("OK Button")) -> (error out=w414:errorcluster)  [unwired: 1 in, 4 out]
              }
            }
          }
          frame #2 {
            w419 = u8 0 ("Disabled")
            n322 = local write "ConnectChannel"(FALSE ("ConnectChannel")) -> ()
            n323 = property on="ConnectAll" class="Bool (strict)"("Disabled"=w419) -> ()  [unwired: 2 in, 2 out]
            n324 = property on="Set Output ON All" class="Bool (strict)"("Disabled"=w419) -> ()  [unwired: 2 in, 2 out]
            n325 = property on="AddChannel" class="Bool (strict)"("Disabled"=w419) -> ()  [unwired: 2 in, 2 out]
            n326 = property on="DisconnectChannel" class="Bool (strict)"("Disabled"=w419) -> ()  [unwired: 2 in, 2 out]
            n327 = property on="ReadFromFile" class="Bool (strict)"("Disabled"=w419) -> ()  [unwired: 2 in, 2 out]
            n328 = property on="ConnectChannel" class="Bool (strict)"("Disabled"=w419) -> ()  [unwired: 2 in, 2 out]
            n329 = property on="DeleteChannel" class="Bool (strict)"("Disabled"=w419) -> ()  [unwired: 2 in, 2 out]
            n330 = property on="WriteToFile" class="Bool (strict)"("Disabled"=w419) -> ()  [unwired: 2 in, 2 out]
            n331 = property on="SetCurrentB" class="Bool (strict)"("Disabled"=w419) -> ()  [unwired: 2 in, 2 out]
            n332 = property on="SetOutputOnB" class="Bool (strict)"("Disabled"=w419) -> ()  [unwired: 2 in, 2 out]
            n333 = property on="SetVoltageB" class="Bool (strict)"("Disabled"=w419) -> ()  [unwired: 2 in, 2 out]
            n334 = property on="SetOutputOffB" class="Bool (strict)"("Disabled"=w419) -> ()  [unwired: 2 in, 2 out]
            n335 = property on="SetVoltageAll" class="Bool (strict)"("Disabled"=w419) -> ()  [unwired: 2 in, 2 out]
            n336 = property on="SetCurrentAll" class="Bool (strict)"("Disabled"=w419) -> ()  [unwired: 2 in, 2 out]
            n337 = property on="DisconnectAll" class="Bool (strict)"("Disabled"=w419) -> ()  [unwired: 2 in, 2 out]
          }
        }
        n338 = Merge Errors(w392) -> (w390:errorcluster)
      }
      event "ConnectAll": Value Change {
        n339 = event-data() -> ()  [unwired: 7 out]
        n340 = flat-sequence {
          tunnel: [w425] -> w422
          tunnel: [w434] -> w423
          tunnel: w422 -> [w434]
          frame #0 {
            w424 = u8 2 ("Disabled")
            n341 = property on="ReadFromFile" class="Bool (strict)"("Disabled"=w424) -> ()  [unwired: 2 in, 2 out]
            n342 = property on="WriteToFile" class="Bool (strict)"("Disabled"=w424) -> ()  [unwired: 2 in, 2 out]
            n343 = property on="ConnectAll" class="Bool (strict)"("Disabled"=w424) -> ()  [unwired: 2 in, 2 out]
            n344 = property on="Set Output ON All" class="Bool (strict)"("Disabled"=w424) -> ()  [unwired: 2 in, 2 out]
            n345 = property on="SetOutputOffB" class="Bool (strict)"("Disabled"=w424) -> ()  [unwired: 2 in, 2 out]
            n346 = property on="AddChannel" class="Bool (strict)"("Disabled"=w424) -> ()  [unwired: 2 in, 2 out]
            n347 = property on="DisconnectChannel" class="Bool (strict)"("Disabled"=w424) -> ()  [unwired: 2 in, 2 out]
            n348 = property on="SetCurrentAll" class="Bool (strict)"("Disabled"=w424) -> ()  [unwired: 2 in, 2 out]
            n349 = property on="SetOutputOnB" class="Bool (strict)"("Disabled"=w424) -> ()  [unwired: 2 in, 2 out]
            n350 = property on="ConnectChannel" class="Bool (strict)"("Disabled"=w424) -> ()  [unwired: 2 in, 2 out]
            n351 = property on="DeleteChannel" class="Bool (strict)"("Disabled"=w424) -> ()  [unwired: 2 in, 2 out]
            n352 = property on="SetCurrentB" class="Bool (strict)"("Disabled"=w424) -> ()  [unwired: 2 in, 2 out]
            n353 = property on="SetVoltageB" class="Bool (strict)"("Disabled"=w424) -> ()  [unwired: 2 in, 2 out]
            n354 = property on="SetVoltageAll" class="Bool (strict)"("Disabled"=w424) -> ()  [unwired: 2 in, 2 out]
            n355 = property on="DisconnectAll" class="Bool (strict)"("Disabled"=w424) -> ()  [unwired: 2 in, 2 out]
          }
          frame #1 {
            n356 = local read "Measure_VI"() -> (w427:refnum<vi>[])
            n357 = Array Size(array=w427) -> (size(s)=w426:i32)
            n358 = for {
              N: w426 -> [_]
              tunnel: [w428] -> w425 mode=indexing
              i -> [w429]
              n359 = local read "Measure_VI"() -> (w432:refnum<vi>[])
              n360 = Index Array(array=w432, index=w429) -> (element=w431:refnum<vi>)
              n361 = invoke class="VI" method="Ctrl Val.Set"(reference=w431, "Control Name"="Connect", "Value"=TRUE ("OK Button")) -> (error out=w428:errorcluster)  [unwired: 2 in, 4 out]
            }
          }
          frame #2 {
            w435 = u8 0 ("Disabled")
            n362 = local write "ConnectAll"(FALSE ("ConnectChannel")) -> ()
            n363 = property on="AddChannel" class="Bool (strict)"("Disabled"=w435) -> ()  [unwired: 2 in, 2 out]
            n364 = property on="DisconnectChannel" class="Bool (strict)"("Disabled"=w435) -> ()  [unwired: 2 in, 2 out]
            n365 = property on="ConnectAll" class="Bool (strict)"("Disabled"=w435) -> ()  [unwired: 2 in, 2 out]
            n366 = property on="Set Output ON All" class="Bool (strict)"("Disabled"=w435) -> ()  [unwired: 2 in, 2 out]
            n367 = property on="SetOutputOffB" class="Bool (strict)"("Disabled"=w435) -> ()  [unwired: 2 in, 2 out]
            n368 = property on="SetCurrentAll" class="Bool (strict)"("Disabled"=w435) -> ()  [unwired: 2 in, 2 out]
            n369 = property on="ConnectChannel" class="Bool (strict)"("Disabled"=w435) -> ()  [unwired: 2 in, 2 out]
            n370 = property on="SetVoltageAll" class="Bool (strict)"("Disabled"=w435) -> ()  [unwired: 2 in, 2 out]
            n371 = property on="SetOutputOnB" class="Bool (strict)"("Disabled"=w435) -> ()  [unwired: 2 in, 2 out]
            n372 = property on="DisconnectAll" class="Bool (strict)"("Disabled"=w435) -> ()  [unwired: 2 in, 2 out]
            n373 = property on="ReadFromFile" class="Bool (strict)"("Disabled"=w435) -> ()  [unwired: 2 in, 2 out]
            n374 = property on="WriteToFile" class="Bool (strict)"("Disabled"=w435) -> ()  [unwired: 2 in, 2 out]
            n375 = property on="SetCurrentB" class="Bool (strict)"("Disabled"=w435) -> ()  [unwired: 2 in, 2 out]
            n376 = property on="SetVoltageB" class="Bool (strict)"("Disabled"=w435) -> ()  [unwired: 2 in, 2 out]
            n377 = property on="DeleteChannel" class="Bool (strict)"("Disabled"=w435) -> ()  [unwired: 2 in, 2 out]
          }
        }
        n378 = Merge Errors(w423) -> (w421:errorcluster)
      }
      event "DisconnectAll": Value Change {
        n379 = event-data() -> ()  [unwired: 7 out]
        n380 = flat-sequence {
          tunnel: [w441] -> w439
          tunnel: [w450] -> w438
          tunnel: w439 -> [w450]
          frame #0 {
            w440 = u8 2 ("Disabled")
            n381 = property on="ReadFromFile" class="Bool (strict)"("Disabled"=w440) -> ()  [unwired: 2 in, 2 out]
            n382 = property on="ConnectAll" class="Bool (strict)"("Disabled"=w440) -> ()  [unwired: 2 in, 2 out]
            n383 = property on="ConnectChannel" class="Bool (strict)"("Disabled"=w440) -> ()  [unwired: 2 in, 2 out]
            n384 = property on="AddChannel" class="Bool (strict)"("Disabled"=w440) -> ()  [unwired: 2 in, 2 out]
            n385 = property on="DisconnectChannel" class="Bool (strict)"("Disabled"=w440) -> ()  [unwired: 2 in, 2 out]
            n386 = property on="Set Output ON All" class="Bool (strict)"("Disabled"=w440) -> ()  [unwired: 2 in, 2 out]
            n387 = property on="WriteToFile" class="Bool (strict)"("Disabled"=w440) -> ()  [unwired: 2 in, 2 out]
            n388 = property on="SetOutputOffB" class="Bool (strict)"("Disabled"=w440) -> ()  [unwired: 2 in, 2 out]
            n389 = property on="SetCurrentAll" class="Bool (strict)"("Disabled"=w440) -> ()  [unwired: 2 in, 2 out]
            n390 = property on="SetOutputOnB" class="Bool (strict)"("Disabled"=w440) -> ()  [unwired: 2 in, 2 out]
            n391 = property on="DeleteChannel" class="Bool (strict)"("Disabled"=w440) -> ()  [unwired: 2 in, 2 out]
            n392 = property on="SetCurrentB" class="Bool (strict)"("Disabled"=w440) -> ()  [unwired: 2 in, 2 out]
            n393 = property on="SetVoltageB" class="Bool (strict)"("Disabled"=w440) -> ()  [unwired: 2 in, 2 out]
            n394 = property on="SetVoltageAll" class="Bool (strict)"("Disabled"=w440) -> ()  [unwired: 2 in, 2 out]
            n395 = property on="DisconnectAll" class="Bool (strict)"("Disabled"=w440) -> ()  [unwired: 2 in, 2 out]
          }
          frame #1 {
            n396 = local read "Measure_VI"() -> (w443:refnum<vi>[])
            n397 = Array Size(array=w443) -> (size(s)=w442:i32)
            n398 = for {
              N: w442 -> [_]
              tunnel: [w444] -> w441 mode=indexing
              i -> [w445]
              n399 = local read "Measure_VI"() -> (w448:refnum<vi>[])
              n400 = Index Array(array=w448, index=w445) -> (element=w447:refnum<vi>)
              n401 = invoke class="VI" method="Ctrl Val.Set"(reference=w447, "Control Name"="Connect", "Value"=FALSE ("OK Button")) -> (error out=w444:errorcluster)  [unwired: 2 in, 4 out]
            }
          }
          frame #2 {
            w451 = u8 0 ("Disabled")
            n402 = local write "DisconnectAll"(FALSE ("ConnectChannel")) -> ()
            n403 = property on="ConnectAll" class="Bool (strict)"("Disabled"=w451) -> ()  [unwired: 2 in, 2 out]
            n404 = property on="ConnectChannel" class="Bool (strict)"("Disabled"=w451) -> ()  [unwired: 2 in, 2 out]
            n405 = property on="AddChannel" class="Bool (strict)"("Disabled"=w451) -> ()  [unwired: 2 in, 2 out]
            n406 = property on="DisconnectChannel" class="Bool (strict)"("Disabled"=w451) -> ()  [unwired: 2 in, 2 out]
            n407 = property on="ReadFromFile" class="Bool (strict)"("Disabled"=w451) -> ()  [unwired: 2 in, 2 out]
            n408 = property on="Set Output ON All" class="Bool (strict)"("Disabled"=w451) -> ()  [unwired: 2 in, 2 out]
            n409 = property on="WriteToFile" class="Bool (strict)"("Disabled"=w451) -> ()  [unwired: 2 in, 2 out]
            n410 = property on="SetOutputOnB" class="Bool (strict)"("Disabled"=w451) -> ()  [unwired: 2 in, 2 out]
            n411 = property on="SetCurrentB" class="Bool (strict)"("Disabled"=w451) -> ()  [unwired: 2 in, 2 out]
            n412 = property on="SetVoltageB" class="Bool (strict)"("Disabled"=w451) -> ()  [unwired: 2 in, 2 out]
            n413 = property on="SetVoltageAll" class="Bool (strict)"("Disabled"=w451) -> ()  [unwired: 2 in, 2 out]
            n414 = property on="DisconnectAll" class="Bool (strict)"("Disabled"=w451) -> ()  [unwired: 2 in, 2 out]
            n415 = property on="DeleteChannel" class="Bool (strict)"("Disabled"=w451) -> ()  [unwired: 2 in, 2 out]
            n416 = property on="SetOutputOffB" class="Bool (strict)"("Disabled"=w451) -> ()  [unwired: 2 in, 2 out]
            n417 = property on="SetCurrentAll" class="Bool (strict)"("Disabled"=w451) -> ()  [unwired: 2 in, 2 out]
          }
        }
        n418 = Merge Errors(w438) -> (w437:errorcluster)
      }
      event "SetVoltageB": Value Change {
        n419 = event-data() -> ()  [unwired: 7 out]
        n420 = local write "SetVoltageB"(FALSE ("ConnectChannel")) -> ()
        n421 = flat-sequence {
          tunnel: [w459] -> w455
          tunnel: [w468] -> w454
          tunnel: w455 -> [w468]
          frame #0 {
            w457 = u8 2 ("Disabled")
            n422 = property on="AddChannel" class="Bool (strict)"("Disabled"=w457) -> ()  [unwired: 2 in, 2 out]
            n423 = property on="Set Output ON All" class="Bool (strict)"("Disabled"=w457) -> ()  [unwired: 2 in, 2 out]
            n424 = property on="ConnectAll" class="Bool (strict)"("Disabled"=w457) -> ()  [unwired: 2 in, 2 out]
            n425 = property on="DisconnectChannel" class="Bool (strict)"("Disabled"=w457) -> ()  [unwired: 2 in, 2 out]
            n426 = property on="ReadFromFile" class="Bool (strict)"("Disabled"=w457) -> ()  [unwired: 2 in, 2 out]
            n427 = property on="ConnectChannel" class="Bool (strict)"("Disabled"=w457) -> ()  [unwired: 2 in, 2 out]
            n428 = property on="DeleteChannel" class="Bool (strict)"("Disabled"=w457) -> ()  [unwired: 2 in, 2 out]
            n429 = property on="WriteToFile" class="Bool (strict)"("Disabled"=w457) -> ()  [unwired: 2 in, 2 out]
            n430 = property on="SetCurrentB" class="Bool (strict)"("Disabled"=w457) -> ()  [unwired: 2 in, 2 out]
            n431 = property on="SetOutputOnB" class="Bool (strict)"("Disabled"=w457) -> ()  [unwired: 2 in, 2 out]
            n432 = property on="SetVoltageB" class="Bool (strict)"("Disabled"=w457) -> ()  [unwired: 2 in, 2 out]
            n433 = property on="SetOutputOffB" class="Bool (strict)"("Disabled"=w457) -> ()  [unwired: 2 in, 2 out]
            n434 = property on="SetVoltageAll" class="Bool (strict)"("Disabled"=w457) -> ()  [unwired: 2 in, 2 out]
            n435 = property on="SetCurrentAll" class="Bool (strict)"("Disabled"=w457) -> ()  [unwired: 2 in, 2 out]
            n436 = property on="DisconnectAll" class="Bool (strict)"("Disabled"=w457) -> ()  [unwired: 2 in, 2 out]
          }
          frame #1 {
            n437 = property on="List of channels" class="MCListbox (strict)"() -> ("Value"=w458:i32)  [unwired: 2 in, 2 out]
            n438 = local read "Measure_VI"() -> (w466:refnum<vi>[])
            n439 = local read "SetVoltage"() -> (w464:dbl)
            n440 = Index Array(array=w466, index=w458) -> (element=w465:refnum<vi>)
            n441 = invoke class="VI" method="Ctrl Val.Set"(reference=w465, "Control Name"="SetVoltage", "Value"=w464) -> (reference out=w461:refnum<vi>, error out=w460:errorcluster)  [unwired: 2 in, 3 out]
            n442 = invoke class="VI" method="Ctrl Val.Set"(reference=w461, error in=w460, "Control Name"="NeedToSetVoltage", "Value"=TRUE ("ConnectChannel")) -> (error out=w459:errorcluster)  [unwired: 1 in, 4 out]
          }
          frame #2 {
            w469 = u8 0 ("Disabled")
            n443 = property on="ConnectAll" class="Bool (strict)"("Disabled"=w469) -> ()  [unwired: 2 in, 2 out]
            n444 = property on="Set Output ON All" class="Bool (strict)"("Disabled"=w469) -> ()  [unwired: 2 in, 2 out]
            n445 = property on="AddChannel" class="Bool (strict)"("Disabled"=w469) -> ()  [unwired: 2 in, 2 out]
            n446 = property on="DisconnectChannel" class="Bool (strict)"("Disabled"=w469) -> ()  [unwired: 2 in, 2 out]
            n447 = property on="ReadFromFile" class="Bool (strict)"("Disabled"=w469) -> ()  [unwired: 2 in, 2 out]
            n448 = property on="ConnectChannel" class="Bool (strict)"("Disabled"=w469) -> ()  [unwired: 2 in, 2 out]
            n449 = property on="DeleteChannel" class="Bool (strict)"("Disabled"=w469) -> ()  [unwired: 2 in, 2 out]
            n450 = property on="SetVoltageAll" class="Bool (strict)"("Disabled"=w469) -> ()  [unwired: 2 in, 2 out]
            n451 = property on="SetCurrentAll" class="Bool (strict)"("Disabled"=w469) -> ()  [unwired: 2 in, 2 out]
            n452 = property on="DisconnectAll" class="Bool (strict)"("Disabled"=w469) -> ()  [unwired: 2 in, 2 out]
            n453 = property on="WriteToFile" class="Bool (strict)"("Disabled"=w469) -> ()  [unwired: 2 in, 2 out]
            n454 = property on="SetCurrentB" class="Bool (strict)"("Disabled"=w469) -> ()  [unwired: 2 in, 2 out]
            n455 = property on="SetOutputOnB" class="Bool (strict)"("Disabled"=w469) -> ()  [unwired: 2 in, 2 out]
            n456 = property on="SetVoltageB" class="Bool (strict)"("Disabled"=w469) -> ()  [unwired: 2 in, 2 out]
            n457 = property on="SetOutputOffB" class="Bool (strict)"("Disabled"=w469) -> ()  [unwired: 2 in, 2 out]
          }
        }
        n458 = Merge Errors(w454) -> (w453:errorcluster)
      }
      event "SetOutputOnB": Value Change {
        n459 = event-data() -> ()  [unwired: 2 out]
        n460 = property on="List of channels" class="MCListbox (strict)"() -> ("Value"=w473:i32)  [unwired: 2 in, 2 out]
        n461 = flat-sequence {
          tunnel: w473 -> [w475]
          tunnel: [w475] -> w472
          tunnel: w472 -> [w482]
          tunnel: [w477] -> w471
          tunnel: [w487] -> w470
          tunnel: w471 -> [w487]
          frame #0 {
            w474 = u8 2 ("Disabled")
            n462 = property on="ConnectAll" class="Bool (strict)"("Disabled"=w474) -> ()  [unwired: 2 in, 2 out]
            n463 = property on="Set Output ON All" class="Bool (strict)"("Disabled"=w474) -> ()  [unwired: 2 in, 2 out]
            n464 = property on="AddChannel" class="Bool (strict)"("Disabled"=w474) -> ()  [unwired: 2 in, 2 out]
            n465 = property on="DisconnectChannel" class="Bool (strict)"("Disabled"=w474) -> ()  [unwired: 2 in, 2 out]
            n466 = property on="ReadFromFile" class="Bool (strict)"("Disabled"=w474) -> ()  [unwired: 2 in, 2 out]
            n467 = property on="ConnectChannel" class="Bool (strict)"("Disabled"=w474) -> ()  [unwired: 2 in, 2 out]
            n468 = property on="DeleteChannel" class="Bool (strict)"("Disabled"=w474) -> ()  [unwired: 2 in, 2 out]
            n469 = property on="WriteToFile" class="Bool (strict)"("Disabled"=w474) -> ()  [unwired: 2 in, 2 out]
            n470 = property on="SetCurrentB" class="Bool (strict)"("Disabled"=w474) -> ()  [unwired: 2 in, 2 out]
            n471 = property on="SetOutputOnB" class="Bool (strict)"("Disabled"=w474) -> ()  [unwired: 2 in, 2 out]
            n472 = property on="SetVoltageB" class="Bool (strict)"("Disabled"=w474) -> ()  [unwired: 2 in, 2 out]
            n473 = property on="SetOutputOffB" class="Bool (strict)"("Disabled"=w474) -> ()  [unwired: 2 in, 2 out]
            n474 = property on="SetVoltageAll" class="Bool (strict)"("Disabled"=w474) -> ()  [unwired: 2 in, 2 out]
            n475 = property on="SetCurrentAll" class="Bool (strict)"("Disabled"=w474) -> ()  [unwired: 2 in, 2 out]
            n476 = property on="DisconnectAll" class="Bool (strict)"("Disabled"=w474) -> ()  [unwired: 2 in, 2 out]
          }
          frame #1 {
            n477 = local write "SetOutputOnB"(FALSE ("ConnectChannel")) -> ()
            n478 = local read "Measure_VI"() -> (w485:refnum<vi>[])
            n479 = Index Array(array=w485, index=w482) -> (element=w484:refnum<vi>)
            n480 = invoke class="VI" method="Ctrl Val.Set"(reference=w484, "Control Name"="SetOutput", "Value"=TRUE ("ConnectChannel")) -> (reference out=w479:refnum<vi>, error out=w478:errorcluster)  [unwired: 2 in, 3 out]
            n481 = invoke class="VI" method="Ctrl Val.Set"(reference=w479, error in=w478, "Control Name"="NeedToSetOutput", "Value"=TRUE ("ConnectChannel")) -> (error out=w477:errorcluster)  [unwired: 1 in, 4 out]
          }
          frame #2 {
            w488 = u8 0 ("Disabled")
            n482 = property on="ConnectAll" class="Bool (strict)"("Disabled"=w488) -> ()  [unwired: 2 in, 2 out]
            n483 = property on="Set Output ON All" class="Bool (strict)"("Disabled"=w488) -> ()  [unwired: 2 in, 2 out]
            n484 = property on="AddChannel" class="Bool (strict)"("Disabled"=w488) -> ()  [unwired: 2 in, 2 out]
            n485 = property on="DisconnectChannel" class="Bool (strict)"("Disabled"=w488) -> ()  [unwired: 2 in, 2 out]
            n486 = property on="ReadFromFile" class="Bool (strict)"("Disabled"=w488) -> ()  [unwired: 2 in, 2 out]
            n487 = property on="ConnectChannel" class="Bool (strict)"("Disabled"=w488) -> ()  [unwired: 2 in, 2 out]
            n488 = property on="DeleteChannel" class="Bool (strict)"("Disabled"=w488) -> ()  [unwired: 2 in, 2 out]
            n489 = property on="SetOutputOffB" class="Bool (strict)"("Disabled"=w488) -> ()  [unwired: 2 in, 2 out]
            n490 = property on="SetVoltageAll" class="Bool (strict)"("Disabled"=w488) -> ()  [unwired: 2 in, 2 out]
            n491 = property on="SetCurrentAll" class="Bool (strict)"("Disabled"=w488) -> ()  [unwired: 2 in, 2 out]
            n492 = property on="DisconnectAll" class="Bool (strict)"("Disabled"=w488) -> ()  [unwired: 2 in, 2 out]
            n493 = property on="WriteToFile" class="Bool (strict)"("Disabled"=w488) -> ()  [unwired: 2 in, 2 out]
            n494 = property on="SetCurrentB" class="Bool (strict)"("Disabled"=w488) -> ()  [unwired: 2 in, 2 out]
            n495 = property on="SetOutputOnB" class="Bool (strict)"("Disabled"=w488) -> ()  [unwired: 2 in, 2 out]
            n496 = property on="SetVoltageB" class="Bool (strict)"("Disabled"=w488) -> ()  [unwired: 2 in, 2 out]
          }
        }
      }
      event "Set Output ON All": Value Change {
        n497 = event-data() -> ("NewVal"=w489:bool)  [unwired: 1 out]
        n498 = flat-sequence {
          tunnel: [w494] -> w490
          tunnel: w489 -> [w494]
          tunnel: [w499] -> w492
          tunnel: w490 -> [w496]
          tunnel: [w510] -> w493
          tunnel: w492 -> [w510]
          frame #0 {
            w495 = u8 2 ("Disabled")
            n499 = property on="AddChannel" class="Bool (strict)"("Disabled"=w495) -> ()  [unwired: 2 in, 2 out]
            n500 = property on="DisconnectChannel" class="Bool (strict)"("Disabled"=w495) -> ()  [unwired: 2 in, 2 out]
            n501 = property on="ConnectAll" class="Bool (strict)"("Disabled"=w495) -> ()  [unwired: 2 in, 2 out]
            n502 = property on="ReadFromFile" class="Bool (strict)"("Disabled"=w495) -> ()  [unwired: 2 in, 2 out]
            n503 = property on="ConnectChannel" class="Bool (strict)"("Disabled"=w495) -> ()  [unwired: 2 in, 2 out]
            n504 = property on="DeleteChannel" class="Bool (strict)"("Disabled"=w495) -> ()  [unwired: 2 in, 2 out]
            n505 = property on="WriteToFile" class="Bool (strict)"("Disabled"=w495) -> ()  [unwired: 2 in, 2 out]
            n506 = property on="SetCurrentB" class="Bool (strict)"("Disabled"=w495) -> ()  [unwired: 2 in, 2 out]
            n507 = property on="SetOutputOnB" class="Bool (strict)"("Disabled"=w495) -> ()  [unwired: 2 in, 2 out]
            n508 = property on="SetVoltageB" class="Bool (strict)"("Disabled"=w495) -> ()  [unwired: 2 in, 2 out]
            n509 = property on="SetOutputOffB" class="Bool (strict)"("Disabled"=w495) -> ()  [unwired: 2 in, 2 out]
            n510 = property on="SetVoltageAll" class="Bool (strict)"("Disabled"=w495) -> ()  [unwired: 2 in, 2 out]
            n511 = property on="SetCurrentAll" class="Bool (strict)"("Disabled"=w495) -> ()  [unwired: 2 in, 2 out]
            n512 = property on="DisconnectAll" class="Bool (strict)"("Disabled"=w495) -> ()  [unwired: 2 in, 2 out]
          }
          frame #1 {
            n513 = local read "Measure_VI"() -> (w498:refnum<vi>[])
            n514 = Array Size(array=w498) -> (size(s)=w497:i32)
            n515 = for {
              N: w497 -> [_]
              tunnel: [w501] -> w499 mode=indexing
              tunnel: w496 -> [w500]
              i -> [w503]
              n516 = local read "Measure_VI"() -> (w508:refnum<vi>[])
              n517 = Index Array(array=w508, index=w503) -> (element=w507:refnum<vi>)
              n518 = invoke class="VI" method="Ctrl Val.Set"(reference=w507, "Control Name"="SetOutput", "Value"=w500) -> (reference out=w504:refnum<vi>, error out=w502:errorcluster)  [unwired: 2 in, 3 out]
              n519 = invoke class="VI" method="Ctrl Val.Set"(reference=w504, error in=w502, "Control Name"="NeedToSetOutput", "Value"=TRUE ("ConnectChannel")) -> (error out=w501:errorcluster)  [unwired: 1 in, 4 out]
            }
          }
          frame #2 {
            w511 = u8 0 ("Disabled")
            n520 = disable-structure shown="Disabled" {
              frame Disabled {
                n521 = local write "Set Output ON All"(FALSE ("ConnectChannel")) -> ()
              }
              frame Enabled {
              }
            }
            n522 = property on="ConnectAll" class="Bool (strict)"("Disabled"=w511) -> ()  [unwired: 2 in, 2 out]
            n523 = property on="Set Output ON All" class="Bool (strict)"("Disabled"=w511) -> ()  [unwired: 2 in, 2 out]
            n524 = property on="AddChannel" class="Bool (strict)"("Disabled"=w511) -> ()  [unwired: 2 in, 2 out]
            n525 = property on="DisconnectChannel" class="Bool (strict)"("Disabled"=w511) -> ()  [unwired: 2 in, 2 out]
            n526 = property on="ReadFromFile" class="Bool (strict)"("Disabled"=w511) -> ()  [unwired: 2 in, 2 out]
            n527 = property on="ConnectChannel" class="Bool (strict)"("Disabled"=w511) -> ()  [unwired: 2 in, 2 out]
            n528 = property on="DeleteChannel" class="Bool (strict)"("Disabled"=w511) -> ()  [unwired: 2 in, 2 out]
            n529 = property on="SetVoltageB" class="Bool (strict)"("Disabled"=w511) -> ()  [unwired: 2 in, 2 out]
            n530 = property on="SetOutputOffB" class="Bool (strict)"("Disabled"=w511) -> ()  [unwired: 2 in, 2 out]
            n531 = property on="SetVoltageAll" class="Bool (strict)"("Disabled"=w511) -> ()  [unwired: 2 in, 2 out]
            n532 = property on="SetCurrentAll" class="Bool (strict)"("Disabled"=w511) -> ()  [unwired: 2 in, 2 out]
            n533 = property on="DisconnectAll" class="Bool (strict)"("Disabled"=w511) -> ()  [unwired: 2 in, 2 out]
            n534 = property on="WriteToFile" class="Bool (strict)"("Disabled"=w511) -> ()  [unwired: 2 in, 2 out]
            n535 = property on="SetCurrentB" class="Bool (strict)"("Disabled"=w511) -> ()  [unwired: 2 in, 2 out]
            n536 = property on="SetOutputOnB" class="Bool (strict)"("Disabled"=w511) -> ()  [unwired: 2 in, 2 out]
          }
        }
        n537 = Merge Errors(w493) -> (w491:errorcluster)
      }
      event "SetOutputOffB": Value Change {
        n538 = event-data() -> ()  [unwired: 7 out]
        n539 = local write "SetOutputOffB"(FALSE ("ConnectChannel")) -> ()
        n540 = property on="List of channels" class="MCListbox (strict)"() -> ("Value"=w517:i32)  [unwired: 2 in, 2 out]
        n541 = flat-sequence {
          tunnel: w517 -> [w519]
          tunnel: [w519] -> w516
          tunnel: w516 -> [w526]
          tunnel: [w520] -> w513
          tunnel: [w530] -> w514
          tunnel: w513 -> [w530]
          frame #0 {
            w518 = u8 2 ("Disabled")
            n542 = property on="ConnectAll" class="Bool (strict)"("Disabled"=w518) -> ()  [unwired: 2 in, 2 out]
            n543 = property on="Set Output ON All" class="Bool (strict)"("Disabled"=w518) -> ()  [unwired: 2 in, 2 out]
            n544 = property on="AddChannel" class="Bool (strict)"("Disabled"=w518) -> ()  [unwired: 2 in, 2 out]
            n545 = property on="DisconnectChannel" class="Bool (strict)"("Disabled"=w518) -> ()  [unwired: 2 in, 2 out]
            n546 = property on="ReadFromFile" class="Bool (strict)"("Disabled"=w518) -> ()  [unwired: 2 in, 2 out]
            n547 = property on="ConnectChannel" class="Bool (strict)"("Disabled"=w518) -> ()  [unwired: 2 in, 2 out]
            n548 = property on="DeleteChannel" class="Bool (strict)"("Disabled"=w518) -> ()  [unwired: 2 in, 2 out]
            n549 = property on="WriteToFile" class="Bool (strict)"("Disabled"=w518) -> ()  [unwired: 2 in, 2 out]
            n550 = property on="SetCurrentB" class="Bool (strict)"("Disabled"=w518) -> ()  [unwired: 2 in, 2 out]
            n551 = property on="SetOutputOnB" class="Bool (strict)"("Disabled"=w518) -> ()  [unwired: 2 in, 2 out]
            n552 = property on="SetVoltageB" class="Bool (strict)"("Disabled"=w518) -> ()  [unwired: 2 in, 2 out]
            n553 = property on="SetOutputOffB" class="Bool (strict)"("Disabled"=w518) -> ()  [unwired: 2 in, 2 out]
            n554 = property on="SetVoltageAll" class="Bool (strict)"("Disabled"=w518) -> ()  [unwired: 2 in, 2 out]
            n555 = property on="SetCurrentAll" class="Bool (strict)"("Disabled"=w518) -> ()  [unwired: 2 in, 2 out]
            n556 = property on="DisconnectAll" class="Bool (strict)"("Disabled"=w518) -> ()  [unwired: 2 in, 2 out]
          }
          frame #1 {
            n557 = local read "Measure_VI"() -> (w528:refnum<vi>[])
            n558 = Index Array(array=w528, index=w526) -> (element=w527:refnum<vi>)
            n559 = invoke class="VI" method="Ctrl Val.Set"(reference=w527, "Control Name"="SetOutput", "Value"=FALSE ("ConnectChannel")) -> (reference out=w523:refnum<vi>, error out=w521:errorcluster)  [unwired: 2 in, 3 out]
            n560 = invoke class="VI" method="Ctrl Val.Set"(reference=w523, error in=w521, "Control Name"="NeedToSetOutput", "Value"=TRUE ("ConnectChannel")) -> (error out=w520:errorcluster)  [unwired: 1 in, 4 out]
          }
          frame #2 {
            w531 = u8 0 ("Disabled")
            n561 = property on="ConnectAll" class="Bool (strict)"("Disabled"=w531) -> ()  [unwired: 2 in, 2 out]
            n562 = property on="Set Output ON All" class="Bool (strict)"("Disabled"=w531) -> ()  [unwired: 2 in, 2 out]
            n563 = property on="AddChannel" class="Bool (strict)"("Disabled"=w531) -> ()  [unwired: 2 in, 2 out]
            n564 = property on="DisconnectChannel" class="Bool (strict)"("Disabled"=w531) -> ()  [unwired: 2 in, 2 out]
            n565 = property on="ReadFromFile" class="Bool (strict)"("Disabled"=w531) -> ()  [unwired: 2 in, 2 out]
            n566 = property on="ConnectChannel" class="Bool (strict)"("Disabled"=w531) -> ()  [unwired: 2 in, 2 out]
            n567 = property on="DeleteChannel" class="Bool (strict)"("Disabled"=w531) -> ()  [unwired: 2 in, 2 out]
            n568 = property on="SetOutputOffB" class="Bool (strict)"("Disabled"=w531) -> ()  [unwired: 2 in, 2 out]
            n569 = property on="SetVoltageAll" class="Bool (strict)"("Disabled"=w531) -> ()  [unwired: 2 in, 2 out]
            n570 = property on="SetCurrentAll" class="Bool (strict)"("Disabled"=w531) -> ()  [unwired: 2 in, 2 out]
            n571 = property on="DisconnectAll" class="Bool (strict)"("Disabled"=w531) -> ()  [unwired: 2 in, 2 out]
            n572 = property on="WriteToFile" class="Bool (strict)"("Disabled"=w531) -> ()  [unwired: 2 in, 2 out]
            n573 = property on="SetCurrentB" class="Bool (strict)"("Disabled"=w531) -> ()  [unwired: 2 in, 2 out]
            n574 = property on="SetOutputOnB" class="Bool (strict)"("Disabled"=w531) -> ()  [unwired: 2 in, 2 out]
            n575 = property on="SetVoltageB" class="Bool (strict)"("Disabled"=w531) -> ()  [unwired: 2 in, 2 out]
          }
        }
      }
      event "WriteToFile": Value Change {
        n576 = event-data() -> ()  [unwired: 7 out]
        n577 = local read "ADRESS"() -> (w536:string[])
        n578 = Array Size(array=w536) -> (size(s)=w535:i32)
        n579 = flat-sequence {
          tunnel: w535 -> [w545]
          tunnel: [w537] -> w533
          tunnel: [w578] -> w534
          tunnel: w533 -> [w578]
          frame #0 {
            n580 = Number To Decimal String(number=w545) -> (decimal integer string=w540:string)  [unwired: 1 out]
            n581 = Write to Text File(text=w540) -> (refnum out=w539:refnum<file>, cancelled=w538:bool, error out=w541:errorcluster)  [unwired: 1 in, 2 out]
            n582 = Write to Text File(file (use dialog)=w539, text="\nИМЯ  АДРЕС  ТОК  НАПРЯЖЕНИЕ", error in=w541) -> (refnum out=w542:refnum<file>, error out=w543:errorcluster)  [unwired: 2 out]
            n583 = for {
              N: w545 -> [_]
              tunnel: w538 -> [w555]
              tunnel: w543 -> [w550]
              tunnel: w542 -> [w557]
              tunnel: [w548] -> w537 mode=indexing
              i -> [w556]
              w561 = "" ("Control Name")
              w567 = "\t"
              n584 = local read "Measure_VI"() -> (w565:refnum<vi>[])
              n585 = Index Array(array=w565, index=w556) -> (element=w564:refnum<vi>)
              n586 = invoke class="VI" method="Ctrl Val.Get"(reference=w564, "Control Name"="SetVoltageStr") -> (reference out=w559:refnum<vi>, error out=w552:errorcluster, "Get Control Value Variant"=w566:variant)  [unwired: 2 in, 1 out]
              n587 = invoke class="VI" method="Ctrl Val.Get"(reference=w559, error in=w552, "Control Name"="SetCurrentStr") -> (error out=w551:errorcluster, "Get Control Value Variant"=w562:variant)  [unwired: 1 in, 2 out]
              n588 = local read "ADRESS"() -> (w572:string[])
              n589 = local read "NAME"() -> (w570:string[])
              n590 = Index Array(array=w570, index=w556) -> (element=w568:string)
              n591 = Index Array(array=w572, index=w556) -> (element=w571:string)
              n592 = Variant To Data(type=w561, Variant=w562) -> (data=w546:string, error out=w554:errorcluster)  [unwired: 1 in]
              n593 = Variant To Data(type=w561, Variant=w566) -> (data=w547:string, error out=w553:errorcluster)  [unwired: 1 in]
              n594 = Merge Errors(w551, w554, w553, w550) -> (w549:errorcluster)
              n595 = Concatenate Strings("\r\n", w568, w567, w571, w567, w546, w567, w547) -> (w558:string)
              n596 = case shown="False" w555 {
                tunnel: w557 -> [w575 _]
                tunnel: w558 -> [w576 _]
                tunnel: w549 -> [w574 w577]
                tunnel: [w573 w577] -> w548
                frame False {
                  n597 = Write to Text File(file (use dialog)=w575, text=w576, error in=w574) -> (error out=w573:errorcluster)  [unwired: 3 out]
                }
                frame True {
                }
              }
            }
          }
          frame #1 {
            n598 = local write "WriteToFile"(FALSE ("ConnectChannel")) -> ()
          }
        }
        n599 = Merge Errors(w534) -> (w532:errorcluster)
      }
      event "ReadFromFile": Value Change {
        n600 = event-data() -> ()  [unwired: 2 out]
        n601 = Read from Text File(count=100) -> (text=w586:string[], cancelled=w585:bool, error out=w584:errorcluster)  [unwired: 1 in, 3 out]
        n602 = local read "ReadFromFile"() -> (w582:bool)
        n603 = Not(x=w585) -> (.not. x?=w581:bool)
        n604 = And(x=w582, y=w581) -> (x .and. y?=w580:bool)
        n605 = case shown="True" w580 {
          tunnel: w586 -> [_ w590]
          tunnel: w584 -> [w588 w592]
          tunnel: [w588 w591] -> w583
          frame False {
            n606 = local write "ReadFromFile"(FALSE ("ConnectChannel")) -> ()
          }
          frame True {
            n607 = flat-sequence {
              tunnel: w592 -> [w599]
              tunnel: [w598] -> w594
              tunnel: w594 -> [w613]
              tunnel: [w613] -> w593
              tunnel: w593 -> [_]
              tunnel: [w622] -> w596
              tunnel: w590 -> [w624]
              tunnel: w596 -> [w658]
              tunnel: [w658] -> w595
              frame #0 {
                w597 = u8 2 ("Disabled")
                n608 = disable-structure shown="Enabled" {
                  disable-tunnel: w599 -> [w602 w611]
                  disable-tunnel: [w601 w611] -> w598
                  frame Disabled {
                    n609 = local read "Measure_VI"() -> (w603:refnum<vi>[])
                    n610 = Array Size(array=w603) -> (size(s)=w600:i32)
                    n611 = for {
                      N: w600 -> [_]
                      tunnel: w603 -> [w607]
                      tunnel: w602 -> [w605]
                      tunnel: [w604] -> w601 mode=indexing
                      i -> [w608]
                      n612 = Index Array(array=w607, index=w608) -> (element=w606:refnum<vi>)
                      n613 = invoke class="VI" method="Ctrl Val.Set"(reference=w606, error in=w605, "Control Name"="Connect", "Value"=FALSE) -> (error out=w604:errorcluster)  [unwired: 1 in, 4 out]
                    }
                  }
                  frame Enabled {
                  }
                }
                n614 = property on="Set Output ON All" class="Bool (strict)"("Disabled"=w597) -> ()  [unwired: 2 in, 2 out]
                n615 = property on="ConnectAll" class="Bool (strict)"("Disabled"=w597) -> ()  [unwired: 2 in, 2 out]
                n616 = property on="ReadFromFile" class="Bool (strict)"("Disabled"=w597) -> ()  [unwired: 2 in, 2 out]
                n617 = property on="ConnectChannel" class="Bool (strict)"("Disabled"=w597) -> ()  [unwired: 2 in, 2 out]
                n618 = property on="DisconnectChannel" class="Bool (strict)"("Disabled"=w597) -> ()  [unwired: 2 in, 2 out]
                n619 = property on="WriteToFile" class="Bool (strict)"("Disabled"=w597) -> ()  [unwired: 2 in, 2 out]
                n620 = property on="AddChannel" class="Bool (strict)"("Disabled"=w597) -> ()  [unwired: 2 in, 2 out]
                n621 = property on="SetOutputOnB" class="Bool (strict)"("Disabled"=w597) -> ()  [unwired: 2 in, 2 out]
                n622 = property on="DeleteChannel" class="Bool (strict)"("Disabled"=w597) -> ()  [unwired: 2 in, 2 out]
                n623 = property on="SetCurrentB" class="Bool (strict)"("Disabled"=w597) -> ()  [unwired: 2 in, 2 out]
                n624 = property on="SetOutputOffB" class="Bool (strict)"("Disabled"=w597) -> ()  [unwired: 2 in, 2 out]
                n625 = property on="SetCurrentAll" class="Bool (strict)"("Disabled"=w597) -> ()  [unwired: 2 in, 2 out]
                n626 = property on="SetVoltageB" class="Bool (strict)"("Disabled"=w597) -> ()  [unwired: 2 in, 2 out]
                n627 = property on="SetVoltageAll" class="Bool (strict)"("Disabled"=w597) -> ()  [unwired: 2 in, 2 out]
                n628 = property on="DisconnectAll" class="Bool (strict)"("Disabled"=w597) -> ()  [unwired: 2 in, 2 out]
              }
              frame #1 {
                n629 = Wait (ms)(milliseconds to wait=u32 1000) -> ()  [unwired: 1 out]
              }
              frame #2 {
                n630 = local read "Measure_VI"() -> (w615:refnum<vi>[])
                n631 = Array Size(array=w615) -> (size(s)=w614:i32)
                n632 = for {
                  N: w614 -> [_]
                  tunnel: w615 -> [w617]
                  i -> [w618]
                  n633 = Index Array(array=w617, index=w618) -> (element=w616:refnum<vi>)
                  n634 = invoke class="VI" method="Abort VI"(reference=w616) -> ()  [unwired: 2 in, 3 out]
                }
              }
              frame #3 {
                w621 = string[] [] ("GlobalInAdress")
                n635 = Wait (ms)(milliseconds to wait=u32 250) -> ()  [unwired: 1 out]
                n636 = local write "NAME"(w621) -> ()
                n637 = local write "ADRESS"(w621) -> ()
                n638 = local write "Measure_VI"(refnum<vi>[] []) -> ()
              }
              frame #4 {
                n639 = Index Array(array=w624, index=0) -> (element=w627:string)
                n640 = Decimal String To Number(string=w627) -> (number=w625:i32)  [unwired: 3 out]
                n641 = for {
                  N: w625 -> [_]
                  tunnel: w624 -> [w652]
                  tunnel: [w630] -> w623 mode=indexing
                  i -> [w655]
                  n642 = Add(x=2, y=w655) -> (x+y=w654:i32)
                  n643 = Index Array(array=w652, index=w654) -> (element=w651:string)
                  n644 = Spreadsheet String To Array(format string="%s", spreadsheet string=w651, array type (2D Dbl)=string[] [] ("GlobalInAdress")) -> (array=w642:string[])  [unwired: 1 out]
                  n645 = Index Array(array=w642, index=2) -> (element=w628:string)
                  n646 = Index Array(array=w642, index=0) -> (element=w646:string)
                  n647 = Index Array(array=w642, index=1) -> (element=w647:string)
                  n648 = Index Array(array=w642, index=3) -> (element=w629:string)
                  n649 = local read "Measure_VI"() -> (w639:refnum<vi>[])
                  n650 = local read "ADRESS"() -> (w640:string[])
                  n651 = Scan From String(input string=w628, default 1=0.0 ("default value 1")) -> (output 1=w635:dbl)  [unwired: 3 in, 3 out]
                  n652 = Scan From String(input string=w629, default 1=0.0 ("default value 1")) -> (output 1=w637:dbl)  [unwired: 3 in, 3 out]
                  n653 = local read "NAME"() -> (w641:string[])
                  n654 = call "AddChannel.vi"("VIRef"=w639, "Name"=w646, "SetCurrent"=w635, "ADRESS"=w640, "NAME"=w641, "Address"=w647, "SetVoltage"=w637) -> ("NAMEOut"=w634:string[], "error out"=w631:errorcluster, "ADRESSOut"=w632:string[], "VIRefOut"=w633:refnum<vi>[])  [unwired: 1 in, 4 out]
                  n655 = local write "NAME"(w634) -> ()
                  n656 = flat-sequence {
                    tunnel: w631 -> [w657]
                    tunnel: [w657] -> w630
                    frame #0 {
                      n657 = Wait (ms)(milliseconds to wait=u32 50) -> ()  [unwired: 1 out]
                    }
                  }
                  n658 = local write "ADRESS"(w632) -> ()
                  n659 = local write "Measure_VI"(w633) -> ()
                }
                n660 = Merge Errors(w623) -> (w622:errorcluster)
              }
              frame #5 {
                w659 = u8 0 ("Disabled")
                n661 = local write "ReadFromFile"(FALSE ("ConnectChannel")) -> ()
                n662 = property on="ConnectAll" class="Bool (strict)"("Disabled"=w659) -> ()  [unwired: 2 in, 2 out]
                n663 = property on="Set Output ON All" class="Bool (strict)"("Disabled"=w659) -> ()  [unwired: 2 in, 2 out]
                n664 = property on="AddChannel" class="Bool (strict)"("Disabled"=w659) -> ()  [unwired: 2 in, 2 out]
                n665 = property on="DisconnectChannel" class="Bool (strict)"("Disabled"=w659) -> ()  [unwired: 2 in, 2 out]
                n666 = property on="ReadFromFile" class="Bool (strict)"("Disabled"=w659) -> ()  [unwired: 2 in, 2 out]
                n667 = property on="ConnectChannel" class="Bool (strict)"("Disabled"=w659) -> ()  [unwired: 2 in, 2 out]
                n668 = property on="DeleteChannel" class="Bool (strict)"("Disabled"=w659) -> ()  [unwired: 2 in, 2 out]
                n669 = property on="WriteToFile" class="Bool (strict)"("Disabled"=w659) -> ()  [unwired: 2 in, 2 out]
                n670 = property on="SetCurrentB" class="Bool (strict)"("Disabled"=w659) -> ()  [unwired: 2 in, 2 out]
                n671 = property on="SetOutputOnB" class="Bool (strict)"("Disabled"=w659) -> ()  [unwired: 2 in, 2 out]
                n672 = property on="SetVoltageB" class="Bool (strict)"("Disabled"=w659) -> ()  [unwired: 2 in, 2 out]
                n673 = property on="SetOutputOffB" class="Bool (strict)"("Disabled"=w659) -> ()  [unwired: 2 in, 2 out]
                n674 = property on="SetVoltageAll" class="Bool (strict)"("Disabled"=w659) -> ()  [unwired: 2 in, 2 out]
                n675 = property on="SetCurrentAll" class="Bool (strict)"("Disabled"=w659) -> ()  [unwired: 2 in, 2 out]
                n676 = property on="DisconnectAll" class="Bool (strict)"("Disabled"=w659) -> ()  [unwired: 2 in, 2 out]
              }
            }
            n677 = Merge Errors(w595) -> (w591:errorcluster)
          }
        }
      }
      event "SetCurrentB": Value Change {
        n678 = event-data() -> ()  [unwired: 7 out]
        n679 = local write "SetCurrentB"(FALSE ("ConnectChannel")) -> ()
        n680 = property on="List of channels" class="MCListbox (strict)"() -> (error out=w663:errorcluster, "Value"=w667:i32)  [unwired: 2 in, 1 out]
        n681 = flat-sequence {
          tunnel: w667 -> [w670]
          tunnel: [w670] -> w666
          tunnel: [w668] -> w664
          tunnel: w663 -> [w668]
          tunnel: w666 -> [w672]
          tunnel: w664 -> [w671]
          tunnel: [w673] -> w662
          tunnel: [w682] -> w661
          tunnel: w662 -> [w682]
          frame #0 {
            w669 = u8 2 ("Disabled")
            n682 = property on="AddChannel" class="Bool (strict)"("Disabled"=w669) -> ()  [unwired: 2 in, 2 out]
            n683 = property on="Set Output ON All" class="Bool (strict)"("Disabled"=w669) -> ()  [unwired: 2 in, 2 out]
            n684 = property on="ConnectAll" class="Bool (strict)"("Disabled"=w669) -> ()  [unwired: 2 in, 2 out]
            n685 = property on="DisconnectChannel" class="Bool (strict)"("Disabled"=w669) -> ()  [unwired: 2 in, 2 out]
            n686 = property on="ReadFromFile" class="Bool (strict)"("Disabled"=w669) -> ()  [unwired: 2 in, 2 out]
            n687 = property on="ConnectChannel" class="Bool (strict)"("Disabled"=w669) -> ()  [unwired: 2 in, 2 out]
            n688 = property on="DeleteChannel" class="Bool (strict)"("Disabled"=w669) -> ()  [unwired: 2 in, 2 out]
            n689 = property on="WriteToFile" class="Bool (strict)"("Disabled"=w669) -> ()  [unwired: 2 in, 2 out]
            n690 = property on="SetCurrentB" class="Bool (strict)"("Disabled"=w669) -> ()  [unwired: 2 in, 2 out]
            n691 = property on="SetOutputOnB" class="Bool (strict)"("Disabled"=w669) -> ()  [unwired: 2 in, 2 out]
            n692 = property on="SetVoltageB" class="Bool (strict)"("Disabled"=w669) -> ()  [unwired: 2 in, 2 out]
            n693 = property on="SetOutputOffB" class="Bool (strict)"("Disabled"=w669) -> ()  [unwired: 2 in, 2 out]
            n694 = property on="SetVoltageAll" class="Bool (strict)"("Disabled"=w669) -> ()  [unwired: 2 in, 2 out]
            n695 = property on="SetCurrentAll" class="Bool (strict)"("Disabled"=w669) -> ()  [unwired: 2 in, 2 out]
            n696 = property on="DisconnectAll" class="Bool (strict)"("Disabled"=w669) -> ()  [unwired: 2 in, 2 out]
          }
          frame #1 {
            n697 = local read "Measure_VI"() -> (w680:refnum<vi>[])
            n698 = local read "SetCurrent"() -> (w678:dbl)
            n699 = Index Array(array=w680, index=w672) -> (element=w679:refnum<vi>)
            n700 = invoke class="VI" method="Ctrl Val.Set"(reference=w679, error in=w671, "Control Name"="SetCurrent", "Value"=w678) -> (reference out=w675:refnum<vi>, error out=w674:errorcluster)  [unwired: 1 in, 3 out]
            n701 = invoke class="VI" method="Ctrl Val.Set"(reference=w675, error in=w674, "Control Name"="NeedToSetCurrent", "Value"=TRUE ("ConnectChannel")) -> (error out=w673:errorcluster)  [unwired: 1 in, 4 out]
          }
          frame #2 {
            w683 = u8 0 ("Disabled")
            n702 = property on="AddChannel" class="Bool (strict)"("Disabled"=w683) -> ()  [unwired: 2 in, 2 out]
            n703 = property on="Set Output ON All" class="Bool (strict)"("Disabled"=w683) -> ()  [unwired: 2 in, 2 out]
            n704 = property on="DisconnectChannel" class="Bool (strict)"("Disabled"=w683) -> ()  [unwired: 2 in, 2 out]
            n705 = property on="ConnectAll" class="Bool (strict)"("Disabled"=w683) -> ()  [unwired: 2 in, 2 out]
            n706 = property on="ReadFromFile" class="Bool (strict)"("Disabled"=w683) -> ()  [unwired: 2 in, 2 out]
            n707 = property on="ConnectChannel" class="Bool (strict)"("Disabled"=w683) -> ()  [unwired: 2 in, 2 out]
            n708 = property on="DeleteChannel" class="Bool (strict)"("Disabled"=w683) -> ()  [unwired: 2 in, 2 out]
            n709 = property on="WriteToFile" class="Bool (strict)"("Disabled"=w683) -> ()  [unwired: 2 in, 2 out]
            n710 = property on="SetCurrentB" class="Bool (strict)"("Disabled"=w683) -> ()  [unwired: 2 in, 2 out]
            n711 = property on="SetOutputOnB" class="Bool (strict)"("Disabled"=w683) -> ()  [unwired: 2 in, 2 out]
            n712 = property on="SetVoltageB" class="Bool (strict)"("Disabled"=w683) -> ()  [unwired: 2 in, 2 out]
            n713 = property on="SetOutputOffB" class="Bool (strict)"("Disabled"=w683) -> ()  [unwired: 2 in, 2 out]
            n714 = property on="SetVoltageAll" class="Bool (strict)"("Disabled"=w683) -> ()  [unwired: 2 in, 2 out]
            n715 = property on="SetCurrentAll" class="Bool (strict)"("Disabled"=w683) -> ()  [unwired: 2 in, 2 out]
            n716 = property on="DisconnectAll" class="Bool (strict)"("Disabled"=w683) -> ()  [unwired: 2 in, 2 out]
          }
        }
      }
      event "DeleteChannel": Value Change {
        n717 = event-data() -> ()  [unwired: 7 out]
        n718 = property on="List of channels" class="MCListbox (strict)"() -> ("Value"=w687:i32)  [unwired: 2 in, 2 out]
        n719 = flat-sequence {
          tunnel: [w696] -> w688
          tunnel: w687 -> [w696]
          tunnel: [w700] -> w695
          tunnel: [w698] -> w694
          tunnel: [w699] -> w693
          tunnel: w688 -> [w698]
          tunnel: [w706] -> w692
          tunnel: w695 -> [w706]
          tunnel: [w705] -> w691
          tunnel: w694 -> [w705]
          tunnel: w693 -> [w704]
          tunnel: [w704] -> w690
          tunnel: w692 -> [w711]
          tunnel: [w710] -> w689
          tunnel: w691 -> [w710]
          tunnel: w690 -> [w709]
          tunnel: [w708] -> w685
          tunnel: w689 -> [w713]
          tunnel: [w712] -> w686
          tunnel: w685 -> [w712]
          tunnel: w686 -> [w721]
          tunnel: [w721] -> w684
          frame #0 {
            w697 = u8 2 ("Disabled")
            n720 = property on="AddChannel" class="Bool (strict)"("Disabled"=w697) -> ()  [unwired: 2 in, 2 out]
            n721 = property on="Set Output ON All" class="Bool (strict)"("Disabled"=w697) -> ()  [unwired: 2 in, 2 out]
            n722 = property on="ConnectAll" class="Bool (strict)"("Disabled"=w697) -> ()  [unwired: 2 in, 2 out]
            n723 = property on="DisconnectChannel" class="Bool (strict)"("Disabled"=w697) -> ()  [unwired: 2 in, 2 out]
            n724 = property on="ReadFromFile" class="Bool (strict)"("Disabled"=w697) -> ()  [unwired: 2 in, 2 out]
            n725 = property on="ConnectChannel" class="Bool (strict)"("Disabled"=w697) -> ()  [unwired: 2 in, 2 out]
            n726 = property on="DeleteChannel" class="Bool (strict)"("Disabled"=w697) -> ()  [unwired: 2 in, 2 out]
            n727 = property on="WriteToFile" class="Bool (strict)"("Disabled"=w697) -> ()  [unwired: 2 in, 2 out]
            n728 = property on="SetCurrentB" class="Bool (strict)"("Disabled"=w697) -> ()  [unwired: 2 in, 2 out]
            n729 = property on="SetOutputOnB" class="Bool (strict)"("Disabled"=w697) -> ()  [unwired: 2 in, 2 out]
            n730 = property on="SetVoltageB" class="Bool (strict)"("Disabled"=w697) -> ()  [unwired: 2 in, 2 out]
            n731 = property on="SetOutputOffB" class="Bool (strict)"("Disabled"=w697) -> ()  [unwired: 2 in, 2 out]
            n732 = property on="SetVoltageAll" class="Bool (strict)"("Disabled"=w697) -> ()  [unwired: 2 in, 2 out]
            n733 = property on="SetCurrentAll" class="Bool (strict)"("Disabled"=w697) -> ()  [unwired: 2 in, 2 out]
            n734 = property on="DisconnectAll" class="Bool (strict)"("Disabled"=w697) -> ()  [unwired: 2 in, 2 out]
          }
          frame #1 {
            n735 = local read "Measure_VI"() -> (w702:refnum<vi>[])
            n736 = Index Array(array=w702, index=w698) -> (element=w700:refnum<vi>)
            n737 = invoke class="VI" method="Ctrl Val.Set"(reference=w700, "Control Name"="Connect", "Value"=FALSE ("OK Button")) -> (error out=w699:errorcluster)  [unwired: 2 in, 4 out]
          }
          frame #2 {
            n738 = Wait (ms)(milliseconds to wait=u32 1000) -> ()  [unwired: 1 out]
          }
          frame #3 {
            n739 = invoke class="VI" method="Abort VI"(reference=w711, error in=w709) -> (error out=w708:errorcluster)  [unwired: 1 in, 2 out]
          }
          frame #4 {
            w714 = 1 ("length")
            n740 = local read "Measure_VI"() -> (w720:refnum<vi>[])
            n741 = local read "ADRESS"() -> (w719:string[])
            n742 = local read "NAME"() -> (w715:string[])
            n743 = Delete From Array(array=w720, length=w714, index=w713) -> (array with subset deleted=w717:refnum<vi>[])  [unwired: 1 out]
            n744 = Delete From Array(array=w719, length=w714, index=w713) -> (array with subset deleted=w718:string[])  [unwired: 1 out]
            n745 = Delete From Array(array=w715, length=w714, index=w713) -> (array with subset deleted=w716:string[])  [unwired: 1 out]
            n746 = local write "ADRESS"(w718) -> ()
            n747 = local write "Measure_VI"(w717) -> ()
            n748 = local write "NAME"(w716) -> ()
          }
          frame #5 {
            w722 = u8 0 ("Disabled")
            n749 = local write "DeleteChannel"(FALSE ("DeleteChannel")) -> ()
            n750 = property on="AddChannel" class="Bool (strict)"("Disabled"=w722) -> ()  [unwired: 2 in, 2 out]
            n751 = property on="DisconnectChannel" class="Bool (strict)"("Disabled"=w722) -> ()  [unwired: 2 in, 2 out]
            n752 = property on="ReadFromFile" class="Bool (strict)"("Disabled"=w722) -> ()  [unwired: 2 in, 2 out]
            n753 = property on="ConnectChannel" class="Bool (strict)"("Disabled"=w722) -> ()  [unwired: 2 in, 2 out]
            n754 = property on="DeleteChannel" class="Bool (strict)"("Disabled"=w722) -> ()  [unwired: 2 in, 2 out]
            n755 = property on="WriteToFile" class="Bool (strict)"("Disabled"=w722) -> ()  [unwired: 2 in, 2 out]
            n756 = property on="Set Output ON All" class="Bool (strict)"("Disabled"=w722) -> ()  [unwired: 2 in, 2 out]
            n757 = property on="SetCurrentB" class="Bool (strict)"("Disabled"=w722) -> ()  [unwired: 2 in, 2 out]
            n758 = property on="ConnectAll" class="Bool (strict)"("Disabled"=w722) -> ()  [unwired: 2 in, 2 out]
            n759 = property on="SetOutputOnB" class="Bool (strict)"("Disabled"=w722) -> ()  [unwired: 2 in, 2 out]
            n760 = property on="SetVoltageB" class="Bool (strict)"("Disabled"=w722) -> ()  [unwired: 2 in, 2 out]
            n761 = property on="SetOutputOffB" class="Bool (strict)"("Disabled"=w722) -> ()  [unwired: 2 in, 2 out]
            n762 = property on="SetVoltageAll" class="Bool (strict)"("Disabled"=w722) -> ()  [unwired: 2 in, 2 out]
            n763 = property on="SetCurrentAll" class="Bool (strict)"("Disabled"=w722) -> ()  [unwired: 2 in, 2 out]
            n764 = property on="DisconnectAll" class="Bool (strict)"("Disabled"=w722) -> ()  [unwired: 2 in, 2 out]
          }
        }
      }
    }
    n765 = call <vilib>:"General Error Handler.vi"("type of dialog (OK msg:1)"=u8 0 ("Disabled"), "error in (no error)"=w192) -> ()  [unwired: 14 out]
    n766 = Wait Until Next ms Multiple(millisecond multiple=u32 20) -> ()  [unwired: 1 out]
  }
  n767 = property on="Set Output ON All" class="Bool (strict)"("Disabled"=w17) -> (error out=w11:errorcluster)  [unwired: 2 in, 1 out]
  n768 = property on="SetCurrentAll" class="Bool (strict)"("Disabled"=w17) -> ()  [unwired: 2 in, 2 out]
  n769 = property on="AddChannel" class="Bool (strict)"("Disabled"=w17) -> ()  [unwired: 2 in, 2 out]
  n770 = property on="AddChannel" class="Bool (strict)"("Disabled"=u8 0) -> ()  [unwired: 2 in, 2 out]
  n771 = local write "текущий ист."(u8 0 ("текущий ист.")) -> ()
  n772 = local write "SetOutputOnB"(w4) -> ()
  n773 = local write "ConnectAll"(w4) -> ()
  n774 = local write "SetOutputOffB"(w4) -> ()
  n775 = local write "DisconnectAll"(w4) -> ()
  n776 = disable-structure shown="Disabled" {
    frame Disabled {
      n777 = call <vilib>:"Application Directory.vi"() -> ("Application Directory"=w741:path)
      n778 = Build Path(base path=w741, name or relative path="BuvConfig.dat") -> (appended path=w738:path)
      n779 = Open/Create/Replace File(file path (use dialog)=w738, operation (0:open)=T2."open") -> (refnum out=w736:refnum<file>, error out=w737:errorcluster)  [unwired: 4 in, 1 out]
      n780 = Read from Text File(file (use dialog)=w736, error in=w737) -> (text=w733:string, error out=w728:errorcluster)  [unwired: 2 in, 2 out]
      n781 = Match Pattern(string=w733, regular expression="Z" ("string")) -> (before substring=w732:string, after substring=w729:string)  [unwired: 1 in, 2 out]
      n782 = Scan From String(input string=w729, error in=w728) -> (error out=w725:errorcluster, output 1=w730:dbl)  [unwired: 3 in, 2 out]
      n783 = local write item#-1(w730) -> ()
      n784 = Scan From String(input string=w732, error in=w725, default 1=u16 0 ("default value 1")) -> (error out=w727:errorcluster, output 1=w735:u16)  [unwired: 2 in, 2 out]
      n785 = local write item#-1(w735) -> ()
      n786 = case shown="No Error" w727 {
        selector: w727 -> [w785 w787]
        tunnel: [TRUE ("LoadPhase") FALSE ("LoadPhase")] -> w726
        tunnel: [w785 w787] -> w724
        frame No Error {
        }
        frame Error {
        }
      }
      "LoadPhase" <- w726
      n787 = while {
        tunnel: w724 -> [w742]
        stop <- FALSE stop-if-true
        n788 = flat-sequence {
          tunnel: [w755] -> w750
          tunnel: [w754] -> w749
          tunnel: w742 -> [w753]
          tunnel: w750 -> [w762]
          tunnel: w749 -> [w761]
          tunnel: [w760] -> w748
          tunnel: [w759] -> w747
          tunnel: w748 -> [w773]
          tunnel: [w772] -> w746
          tunnel: w747 -> [w771]
          tunnel: [w770] -> w745
          tunnel: w746 -> [w776]
          tunnel: w745 -> [w775]
          tunnel: [_] -> w744
          tunnel: [_] -> w743
          tunnel: w744 -> [w783]
          tunnel: w743 -> [w780]
          frame #0 {
            n789 = TCP Open Connection(address="172.16.21.81", remote port or service name=u16 4001, timeout ms (60000)=1000, error in (no error)=w753) -> (connection ID=w754:refnum<k5>, error out=w755:errorcluster)  [unwired: 1 in]
            "Buv con ID" <- w754
          }
          frame #1 {
            n790 = case shown="No Error" w762 {
              selector: w762 -> [w763 w769]
              tunnel: w761 -> [w764 w768]
              tunnel: [_ w769] -> w760
              tunnel: [_ w768] -> w759
              frame No Error {
                n791 = local read item#-1() -> (w766)
                n792 = Or(y=w766) -> (x .or. y?=w765:bool)  [unwired: 1 in]
                n793 = case shown="True" w765 {
                  tunnel: w764 -> [_ _]
                  tunnel: w763 -> [_ _]
                  frame False {
                  }
                  frame True {
                    # "Установка опорного напряжения"
                    n794 = local write item#-1(FALSE ("LoadPhase")) -> ()
                  }
                }
              }
              frame Error {
              }
            }
          }
          frame #2 {
          }
          frame #3 {
            n795 = case shown="Error" w776 {
              selector: w776 -> [_ w778]
              tunnel: w775 -> [_ w777]
              tunnel: [_ "*"] -> _
              tunnel: [_ w778] -> w774
              tunnel: [_ w777] -> _
              frame No Error {
              }
              frame Error {
              }
            }
          }
          frame #4 {
            n796 = case shown="Error" w780 {
              frame No Error {
              }
              frame Error {
                w784 = TRUE ("LoadPhase")
                n797 = local write "LoadPhase"(w784) -> ()
                n798 = local write item#-1(w784) -> ()
              }
            }
            n799 = TCP Close Connection(connection ID=w783) -> (error out=w782:errorcluster)  [unwired: 2 in, 1 out]
            n800 = call <vilib>:"General Error Handler.vi"("type of dialog (OK msg:1)"=0 ("milliseconds to wait"), "error in (no error)"=w782) -> ()  [unwired: 9 in, 5 out]
          }
        }
        n801 = Wait Until Next ms Multiple(millisecond multiple=u32 70) -> ()  [unwired: 1 out]
      }
    }
    frame Enabled {
    }
  }
  n802 = property on="DisconnectAll" class="Bool (strict)"(error in=w11, "Disabled"=w17) -> (error out=w10:errorcluster)  [unwired: 1 in, 1 out]
  n803 = property on="DisconnectChannel" class="Bool (strict)"("Disabled"=w17) -> (error out=w16:errorcluster)  [unwired: 2 in, 1 out]
  n804 = property on="WriteToFile" class="Bool (strict)"(error in=w10, "Disabled"=w17) -> (error out=w9:errorcluster)  [unwired: 1 in, 1 out]
  n805 = property on="SetCurrentB" class="Bool (strict)"(error in=w9, "Disabled"=w17) -> ()  [unwired: 1 in, 2 out]
  n806 = property on="ConnectAll" class="Bool (strict)"(error in=w16, "Disabled"=w17) -> (error out=w15:errorcluster)  [unwired: 1 in, 1 out]
  n807 = property on="ReadFromFile" class="Bool (strict)"(error in=w15, "Disabled"=w17) -> (error out=w14:errorcluster)  [unwired: 1 in, 1 out]
  n808 = property on="SetOutputOnB" class="Bool (strict)"("Disabled"=w17) -> (error out=w8:errorcluster)  [unwired: 2 in, 1 out]
  n809 = property on="ConnectChannel" class="Bool (strict)"(error in=w14, "Disabled"=w17) -> (error out=w13:errorcluster)  [unwired: 1 in, 1 out]
  n810 = property on="SetVoltageB" class="Bool (strict)"(error in=w8, "Disabled"=w17) -> (error out=w7:errorcluster)  [unwired: 1 in, 1 out]
  n811 = property on="SetOutputOffB" class="Bool (strict)"(error in=w7, "Disabled"=w17) -> ()  [unwired: 1 in, 2 out]
  n812 = property on="DeleteChannel" class="Bool (strict)"(error in=w13, "Disabled"=w17) -> (error out=w12:errorcluster)  [unwired: 1 in, 1 out]
  n813 = property on="SetVoltageAll" class="Bool (strict)"(error in=w12, "Disabled"=w17) -> ()  [unwired: 1 in, 2 out]
  n814 = event shown="[0] \"stop\": Value Change" {
    selector: _ -> [_]
    dyn-events: _ -> [_]
    timeout: _ -> [_]
    event "stop": Value Change {
      n815 = event-data() -> ()  [unwired: 1 in, 6 out]
      n816 = flat-sequence {
        frame #0 {
          w792 = T3 0 items=["no dialog", "OK message", "continue or stop message", "OK message + warnings", "continue/stop + warnings"] ("type of dialog (OK msg:1)")
          n817 = local read "Measure_VI"() -> (w790:refnum<vi>[])
          n818 = Array Size(array=w790) -> (size(s)=w791:i32)
          n819 = for {
            N: w791 -> [_]
            tunnel: [w804] -> w789 mode=indexing
            tunnel: w790 -> [w803]
            i -> [w805]
            n820 = Index Array(array=w803, index=w805) -> (element=w797:refnum<vi>)
            n821 = To Variant(anything=TRUE ("ConnectChannel")) -> (Variant=w800:variant)
            n822 = invoke on="Invoke Node" class="VI" method="Ctrl Val.Set"(reference=w797, "Control Name"="TCP disconnect", "Value"=w800) -> (reference out=w799:refnum<vi>, error out=w798:errorcluster)  [unwired: 2 in, 3 out]
            n823 = flat-sequence {
              tunnel: [w808] -> w796
              tunnel: w799 -> [w808]
              tunnel: [w807] -> w795
              tunnel: w798 -> [w807]
              frame #0 {
                n824 = Wait (ms)(milliseconds to wait=u32 100) -> ()  [unwired: 1 out]
              }
            }
            n825 = invoke class="VI" method="Abort VI"(reference=w796, error in=w795) -> (error out=w804:errorcluster)  [unwired: 1 in, 2 out]
          }
          n826 = disable-structure shown="Disabled" {
            disable-tunnel: [w810 _] -> w794
            frame Disabled {
              n827 = local read "Measure_VI"() -> (w809:refnum<vi>[])
              n828 = Array Size(array=w809) -> (size(s)=w811:i32)
              n829 = for {
                N: w811 -> [_]
                tunnel: [w813] -> w810 mode=indexing
                tunnel: w809 -> [w812]
                i -> [w814]
                n830 = Index Array(array=w812, index=w814) -> (element=w816:refnum<vi>)
                n831 = invoke class="VI" method="Ctrl Val.Set"(reference=w816, "Control Name"="Connect", "Value"=FALSE ("OK Button")) -> (error out=w813:errorcluster)  [unwired: 2 in, 4 out]
              }
            }
            frame Enabled {
            }
          }
          n832 = Merge Errors(w789, w794) -> (w793:errorcluster)
          n833 = call <vilib>:"General Error Handler.vi"("type of dialog (OK msg:1)"=w792, "error in (no error)"=w793) -> ()  [unwired: 9 in, 5 out]
        }
        frame #1 {
          n834 = Wait (ms)(milliseconds to wait=u32 200) -> ()  [unwired: 1 out]
        }
        frame #2 {
          n835 = Stop(stop? (T)=TRUE) -> ()
        }
      }
    }
  }
  n836 = for "инициализация цветов и размера ячеек табл." {
    N: 50 -> [_]
    i -> [w822]
    # "Линзы пост. тока"
    n837 = flat-sequence {
      tunnel: w822 -> [w827]
      tunnel: [w827] -> w821
      tunnel: w821 -> [w866]
      tunnel: [w866] -> w820
      tunnel: w820 -> [w879]
      frame #0 {
        w823 = "Application font" ("Font Name")
        n838 = Bundle(w827, 4) -> (w839:cluster{i32, i32})  [unwired: 1 in]
        n839 = property on="active" class="MCListbox (strict)"("ActiveCell"=w839, "Height"=u32 35 ("Active Cell:Cell Size:Height"), "CellFontSize"=u16 28 ("Size")) -> ()  [unwired: 2 in, 2 out]
        n840 = Bundle(w827, 0) -> (w850:cluster{i32, i32})  [unwired: 1 in]
        n841 = Bundle(w827, 2) -> (w826:cluster{i32, i32})  [unwired: 1 in]
        n842 = Bundle(w827, 3) -> (w840:cluster{i32, i32})  [unwired: 1 in]
        n843 = Bundle(w827, 1) -> (w849:cluster{i32, i32})  [unwired: 1 in]
        n844 = Bundle(w827, 6) -> (w825:cluster{i32, i32})  [unwired: 1 in]
        n845 = Bundle(w827, 5) -> (w824:cluster{i32, i32})  [unwired: 1 in]
        n846 = property on="active" class="MCListbox (strict)"("ActiveCell"=w850, "Height"=u32 35 ("Active Cell:Cell Size:Height"), "CellFontSize"=u16 28 ("Size"), "CellFontName"=w823) -> ()  [unwired: 2 in, 2 out]
        n847 = property on="active" class="MCListbox (strict)"("ActiveCell"=w826, "Height"=u32 35 ("Active Cell:Cell Size:Height"), "CellFontSize"=u16 28 ("Size"), "CellFontName"=w823) -> ()  [unwired: 2 in, 2 out]
        n848 = property on="active" class="MCListbox (strict)"("ActiveCell"=w840, "Height"=u32 35 ("Active Cell:Cell Size:Height"), "CellFontSize"=u16 28 ("Size"), "CellFontName"=w823) -> ()  [unwired: 2 in, 2 out]
        n849 = property on="active" class="MCListbox (strict)"("ActiveCell"=w849, "Height"=u32 35 ("Active Cell:Cell Size:Height"), "CellFontSize"=u16 28 ("Size"), "CellFontName"=w823) -> ()  [unwired: 2 in, 2 out]
        n850 = property on="active" class="MCListbox (strict)"("ActiveCell"=w825, "Height"=u32 35 ("Active Cell:Cell Size:Height"), "CellFontSize"=u16 28 ("Size"), "CellFontName"=w823) -> ()  [unwired: 2 in, 2 out]
        n851 = property on="active" class="MCListbox (strict)"("ActiveCell"=w824, "Height"=u32 35 ("Active Cell:Cell Size:Height"), "CellFontSize"=u16 28 ("Size"), "CellFontName"=w823) -> ()  [unwired: 2 in, 2 out]
      }
      frame #1 {
        w862 = T4 {"Font Name"="Application font", "Size"=28, "Bold"=FALSE, "Italic"=FALSE, "Underline"=FALSE, "Strikeout"=FALSE, "Color"=6908265} ("Active Cell:Cell Font")
        w857 = T4 {"Font Name"="Application font", "Size"=30, "Bold"=TRUE, "Italic"=FALSE, "Underline"=FALSE, "Strikeout"=FALSE, "Color"=2263842} ("Active Cell:Cell Font")
        n852 = Bundle(w866, 3) -> (w853:cluster{i32, i32})  [unwired: 1 in]
        n853 = Bundle(w866, 2) -> (w856:cluster{i32, i32})  [unwired: 1 in]
        n854 = Bundle(w866, 0) -> (w864:cluster{i32, i32})  [unwired: 1 in]
        n855 = Bundle(w866, 5) -> (w860:cluster{i32, i32})  [unwired: 1 in]
        n856 = Bundle(w866, 4) -> (w859:cluster{i32, i32})  [unwired: 1 in]
        n857 = property on="active" class="MCListbox (strict)"("ActiveCell"=w853, "CellFont"=w857) -> ()  [unwired: 2 in, 2 out]
        n858 = property on="active" class="MCListbox (strict)"("ActiveCell"=w856, "CellFont"=w857) -> ()  [unwired: 2 in, 2 out]
        n859 = property on="active" class="MCListbox (strict)"("ActiveCell"=w864, "CellFont"=T4 {"Font Name"="Application font", "Size"=28, "Bold"=FALSE, "Italic"=FALSE, "Underline"=FALSE, "Strikeout"=FALSE, "Color"=0} ("Active Cell:Cell Font")) -> ()  [unwired: 2 in, 2 out]
        n860 = property on="active" class="MCListbox (strict)"("ActiveCell"=w860, "CellFont"=w862) -> ()  [unwired: 2 in, 2 out]
        n861 = property on="active" class="MCListbox (strict)"("ActiveCell"=w859, "CellFont"=w862) -> ()  [unwired: 2 in, 2 out]
      }
      frame #2 {
        w878 = T4 {"Font Name"="Application font", "Size"=28, "Bold"=FALSE, "Italic"=FALSE, "Underline"=FALSE, "Strikeout"=FALSE, "Color"=0} ("Active Cell:Cell Font")
        n862 = Bundle(w879, 6) -> (w873:cluster{i32, i32})  [unwired: 1 in]
        n863 = Bundle(w879, 8) -> (w874:cluster{i32, i32})  [unwired: 1 in]
        n864 = Bundle(w879, 7) -> (w875:cluster{i32, i32})  [unwired: 1 in]
        n865 = property on="active" class="MCListbox (strict)"("ActiveCell"=w873, "CellBG"=u32 16777225) -> (error out=w872:errorcluster)  [unwired: 2 in, 1 out]
        n866 = property on="error" class="MCListbox (strict)"("ActiveCell"=w874, "CellBG"=u32 16777225) -> ()  [unwired: 2 in, 2 out]
        n867 = property on="out" class="MCListbox (strict)"("ActiveCell"=w875, "CellBG"=u32 16777225) -> (error out=w876:errorcluster)  [unwired: 2 in, 1 out]
        n868 = property on="active" class="MCListbox (strict)"(error in=w872, "ActiveCell"=w873, "CellFont"=w878) -> ()  [unwired: 1 in, 2 out]
        n869 = property on="active" class="MCListbox (strict)"(error in=w876, "ActiveCell"=w875, "CellFont"=w878) -> ()  [unwired: 1 in, 2 out]
      }
    }
  }
  n870 = Build Array(w1, w1, w1, w1, w1, w1, w1, w1) -> (w2:string[][])
  n871 = Transpose 2D Array(2D array=w2) -> (transposed array=w3:string[][])
  n872 = property on="List of channels" class="MCListbox (strict)"("ItemNames"=w3) -> ()  [unwired: 2 in, 2 out]
  "Measure_VI" <- refnum<vi>[] []
  "ADRESS" <- string[] [] ("GlobalInAdress")
  "NAME" <- string[] [] ("GlobalInAdress")
  "CURRENTSET" <- dbl[] [] ("GlobalInAdress")
